vi "Pick&Place_ladder_shih_v6_center.vi"() -> ()   [LabVIEW 2016]
uses:
  WTF is this.ctl
  Classes/Controllers/I-O/Copy of NI-DAQ Folder/NI-DAQ.lvclass
  D:/INTT/V1/Classes/Controllers/I-O/Copy of I-O Folder/I-O.lvclass
  Classes/Controllers/Dispenser/Copy of Ultimus V2 Folder/Ultimus V2.lvclass
  <vilib>/Analysis/coordinate.llb/2D Cartesian Coordinate Rotation (Scalar).vi
  <vilib>/Utility/file.llb/Read Delimited Spreadsheet (DBL).vi
  <vilib>/Utility/file.llb/Write Delimited Spreadsheet (DBL).vi
  Classes/Controllers/Motion/Copy of Motion Folder/Motion.lvclass
  Classes/Controllers/Camera/Copy of Controller Folder/Controller.lvclass
  <vilib>/Analysis/NI_AALPro.lvlib
  Classes/Controllers/I-O/Copy of I-O Folder/I-O.lvclass
panel:
  in  "offset":dbl[][](array[numeric])=[[0.0, 0.0, 0.0, 0.0], [0.0, 0.0, 0.0, 0.0]]
  out "HPoS_CT":dbl[][](array[numeric]) format="%#_8g"
  out "chip distance by OGP":dbl format="%#_8g"
  out "displacement":dbl[](array[numeric])
  out "gantry position test":dbl[](array[numeric])
  out "stave target position":dbl[](array[numeric])
  out "chip distance by gantry":dbl format="%#_8g"
  out "after SL":dbl[](array[numeric]) format="%#_8g"
  out "after SR":dbl[](array[numeric]) format="%#_8g"
  out "after NL":dbl[](array[numeric]) format="%#_8g"
  out "S chip":dbl[](array[numeric]) format="%#_8g"
  out "N chip":dbl[](array[numeric]) format="%#_8g"
  in  "file path (dialog if empty) 2":path=path "C:/Users/PAGANIS/Desktop/shih cheng wei/OGP/test1-2.txt"
  out "bless from OGP !!! Center of  stave":dbl[](array[numeric])
  out "bless from OGP !! measured stave size":dbl[](array[numeric])
  in  "Bless from OGP":bool
  out "FROM Detail !!! Center of module on stave":dbl[](array[numeric])
  out "FROM Detail !! measured stave size":dbl[](array[numeric])
  in  "Align Stave in detail":bool
  in  "check height?":bool
  in  "Uttimus presssure":i64=10
  out "Status":bool
  out "measured HDI top-left position":dbl[][](array[numeric])
  in  "HDI vacuum channel":i32=18
  in  "vacuum":bool=TRUE
  in  "HDI vacuum":bool
  out "measured stave size":dbl[](array[numeric])
  out "Stave mark":dbl[][](array[numeric])
  out "Center of module on stave":dbl[](array[numeric])
  out "Center of HDI from alignment mark":dbl[](array[numeric])
  out "Measured HDI size":dbl[][](array[numeric])
  out "module positions on stave":T1[][](array[typedef])
  in  "Default Stave dimension":dbl[](array[numeric])=[34.0, 472.0, -0.335295, -0.000320234]
  in  "Default Stave upper left mark":dbl[](array[numeric])=[584.376, 675.576, 70.9882, 0.000840064]
  out "Needle parking position":dbl[](array[numeric])
  in  "Uppler / Lower Stave":bool=TRUE
  out "Gantry current position":dbl[](array[numeric])
  in  "READ Position":bool
  in  "Needle Height Compenstation\n(glue gap)":dbl=0.33
  in  "Needle Alignment":bool
  in  "Parking position":dbl[](array[numeric])=[625.0, 625.0, 0.0, 0.01]
  in  "GOTO":bool
  in  "Default Pickup Tool Position":dbl[][](array[numeric])=[[152.226, 682.729, 36.8129, -0.0151898], [700.0, 800.0, 20.0, 0.01]]
  in  "Number of module \nto be assembled":i32=1
  in  "Default HDI alignment \nmark position":dbl[](array[numeric])=[448.322, 976.582, 74.9872, 0.000191129]
  in  "Default HDI size":dbl[](array[numeric])=[24.2437, 231.446, -0.099339, 0.000191129]
  out "# of tasks excuted":i32
  out "HDI center positions":dbl[][](array[numeric])
  out "PickupTool \nCenterPosition":dbl[](array[numeric])
  in  "Inititalize":bool
  in  "Pick and place":bool
  in  "Deposit Glue":bool
  in  "Measure Pickup Tools":bool
  in  "Align Stave":bool
  out "default module position on stave":dbl[][](array[numeric])
  in  "Stop":bool
  in  "Measure HDI":bool
  # "Ladder Assembly"
  # "Lower\nmodule"
  # "Upper\nmodule"
  # "+"
  # "="
  # "Sensor 0.32 -> 200 micron glue thickness\nChips 0.37-> 140 micron glue thickness"
  # "ACTIONS"
  # "Stave infomation"
  # "theta had *-1"
  # "Module infomation"
  # "Pick and Place"
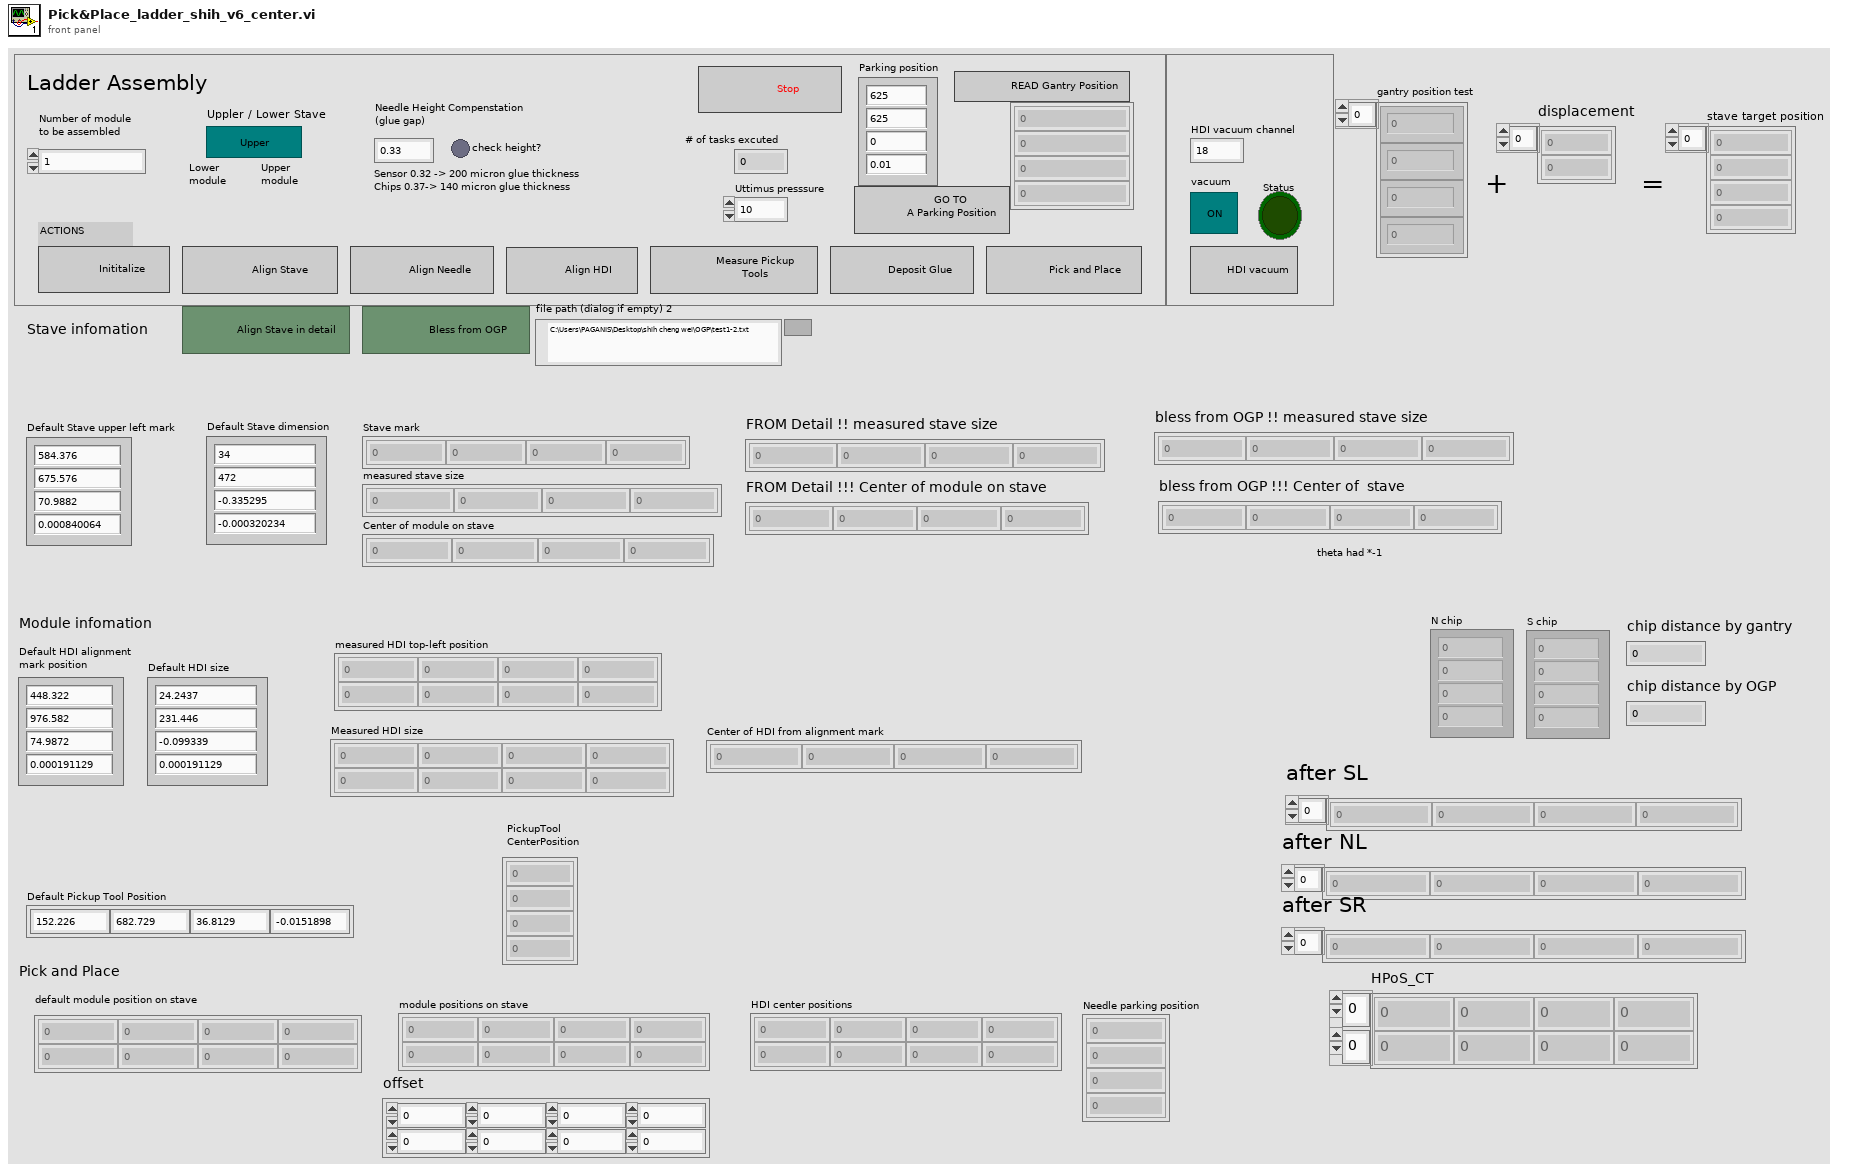
[diagram p1: front panel]
types:
  T1 = typedef "WTF is this.ctl" = dbl
  T2 = typedef "Controller.lvclass/Controllers.ctl" = cluster{"Copy of Motion.lvclass":refnum<class "Motion.lvclass">, "Copy of I-O.lvclass":refnum<class "I-O.lvclass">, "Copy of Dispenser.lvclass":refnum<class "Dispenser.lvclass">}
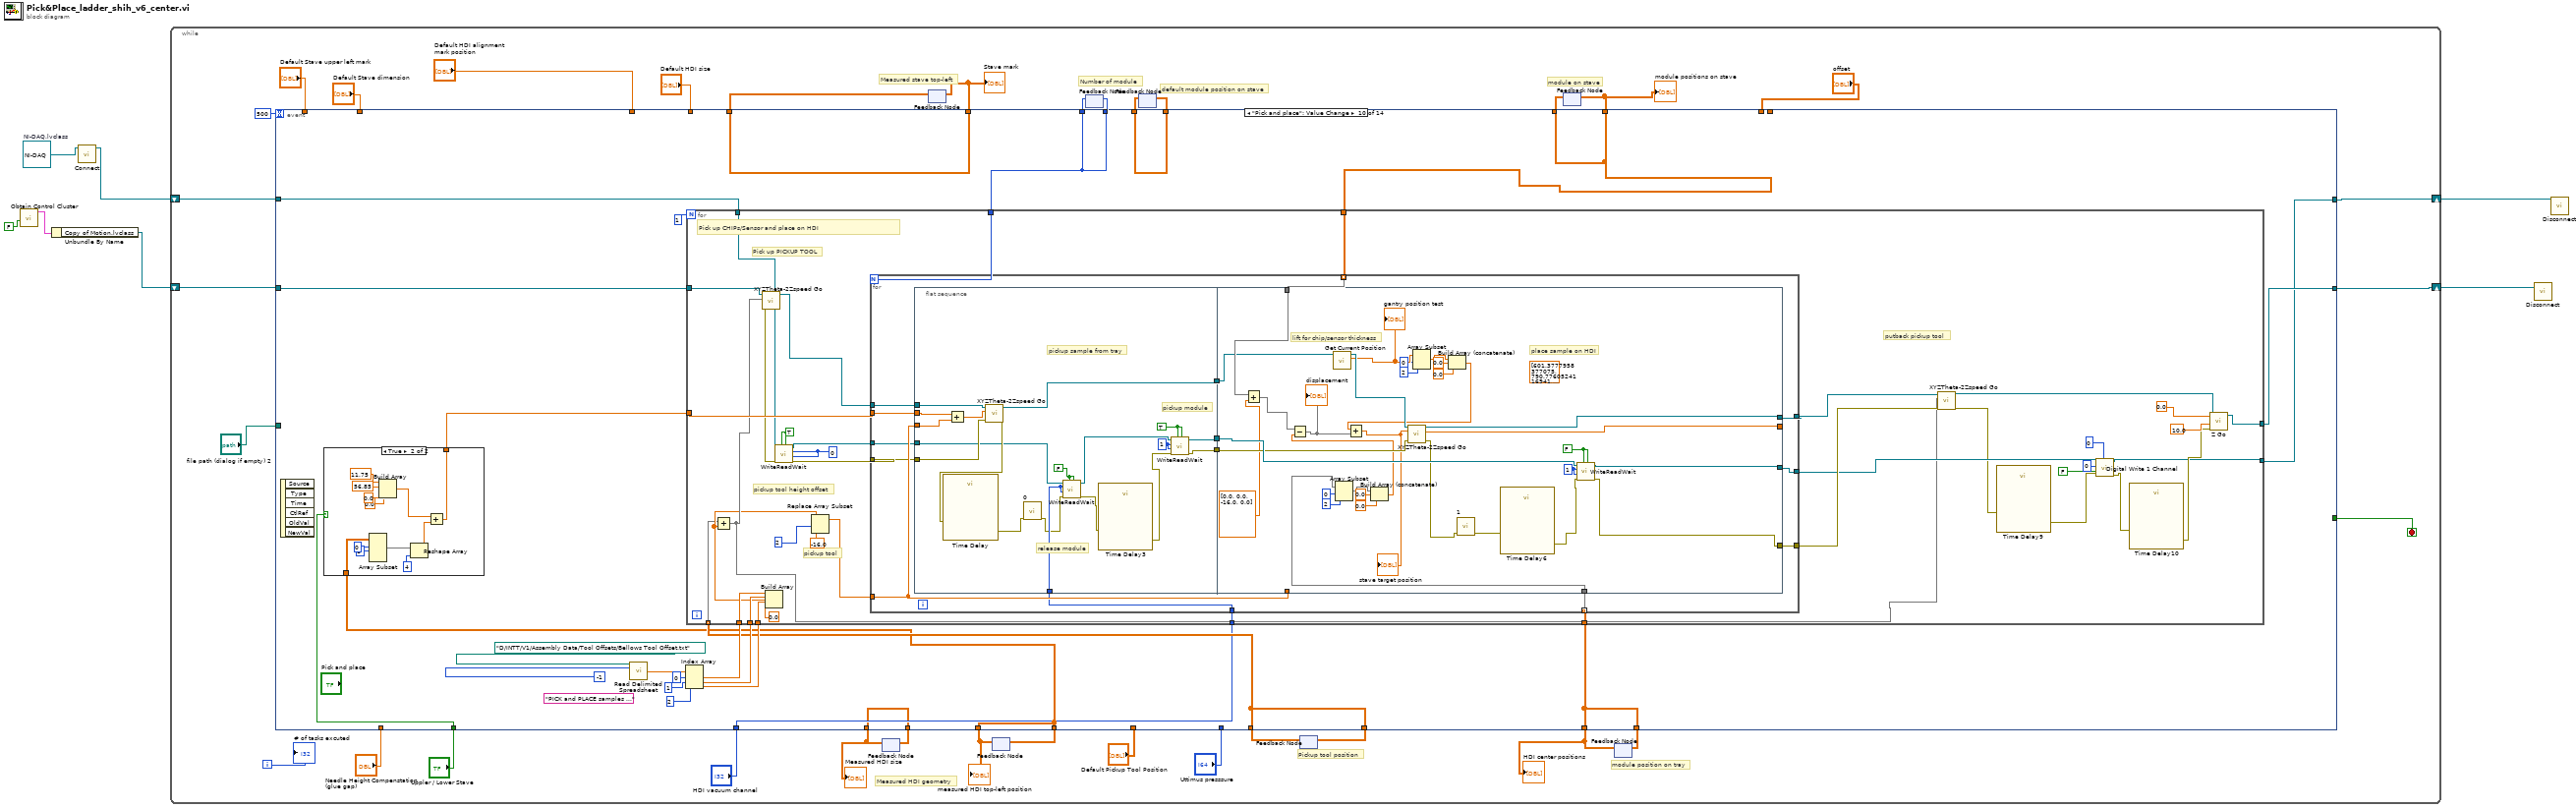
[diagram p0: block diagram]
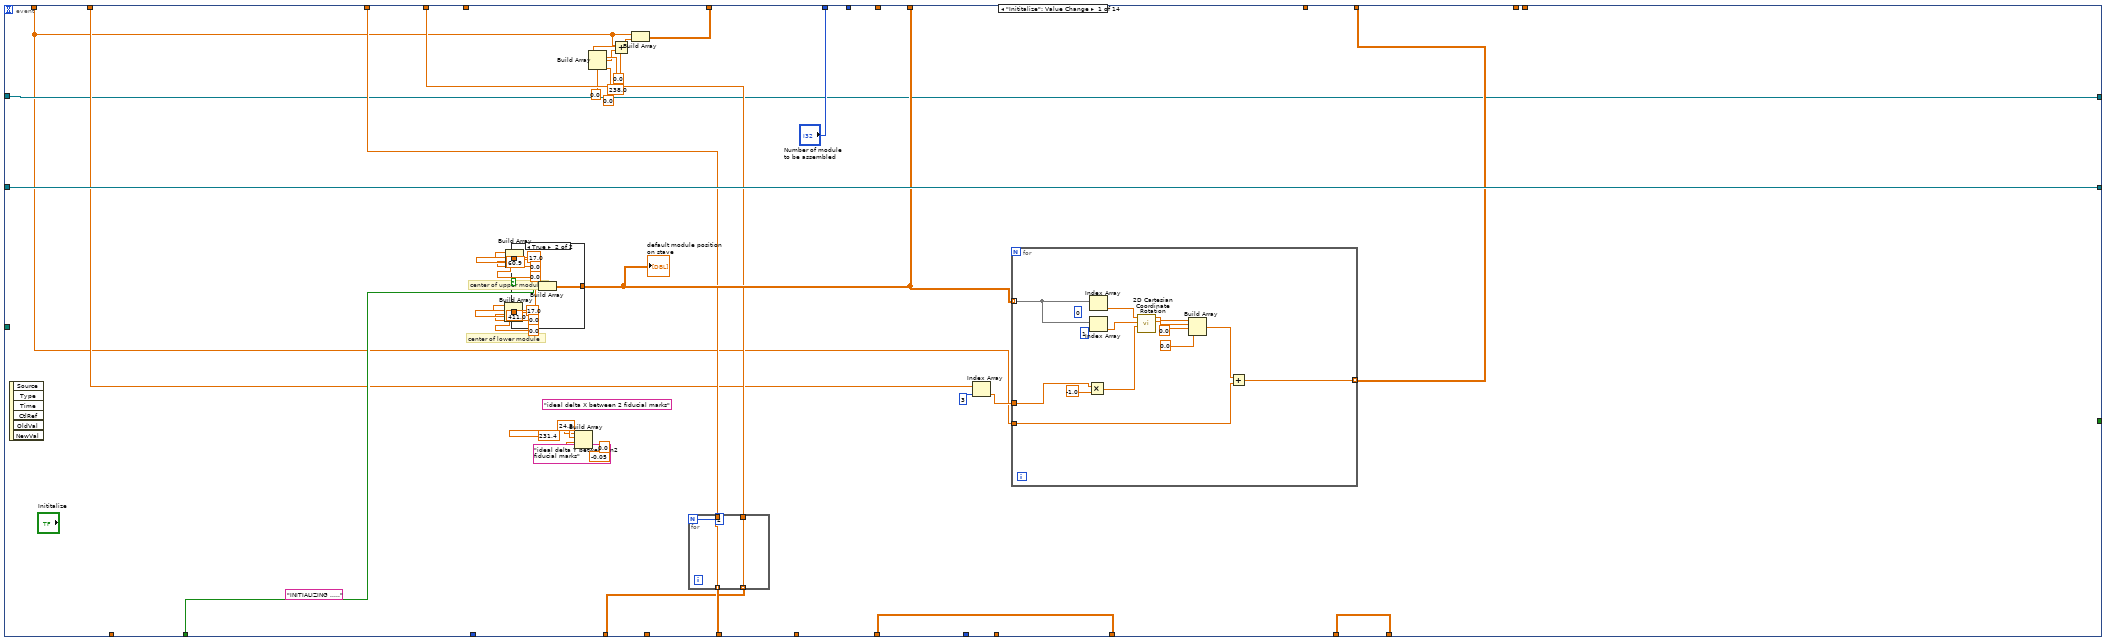
[diagram p2: hidden frame]
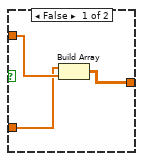
[diagram p3: hidden frame]
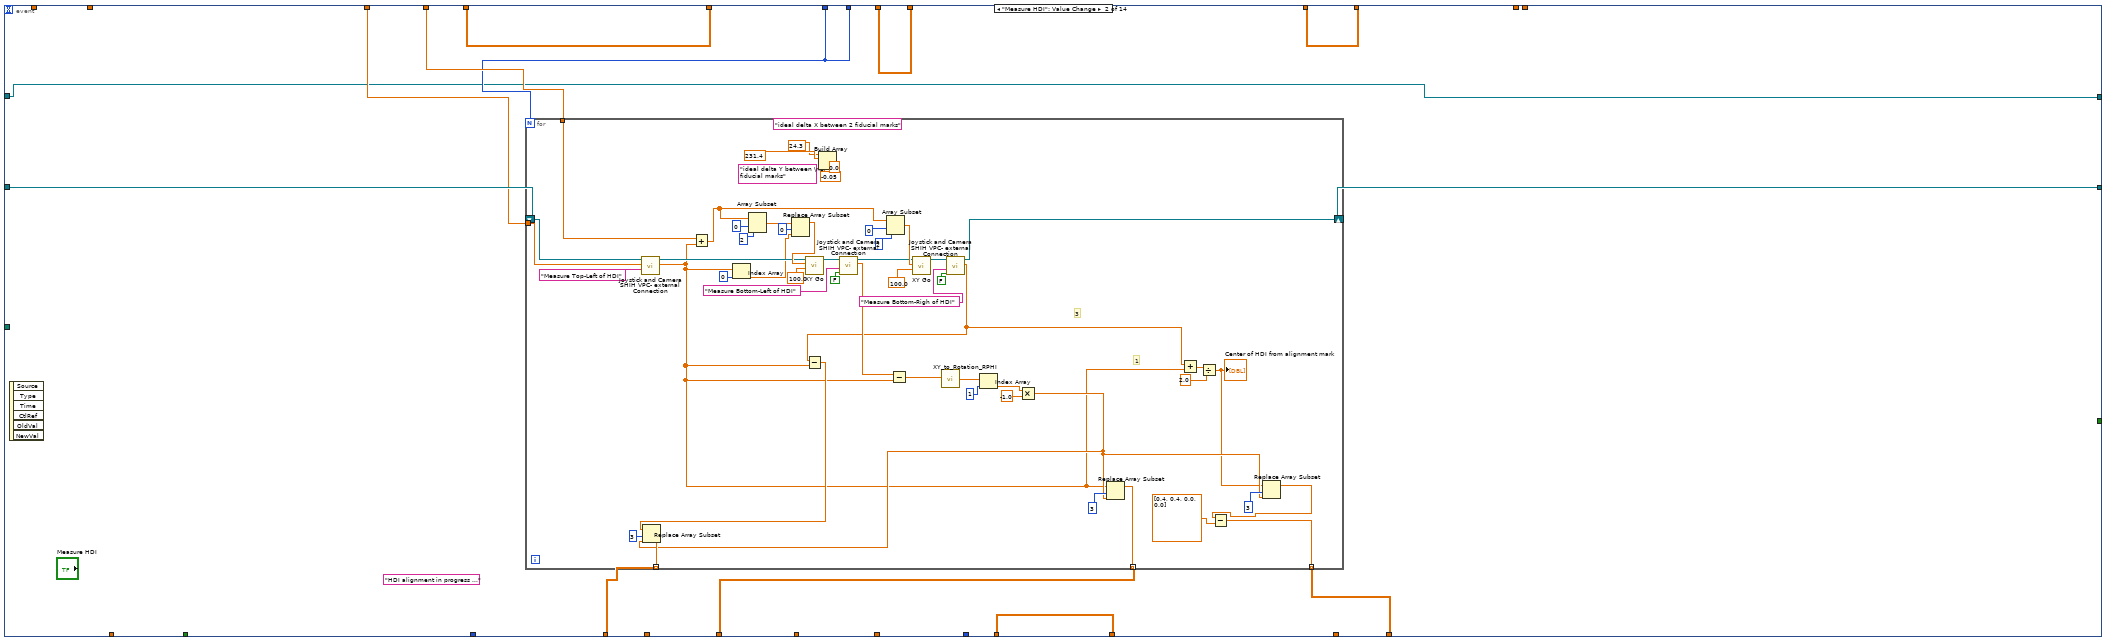
[diagram p4: hidden frame]
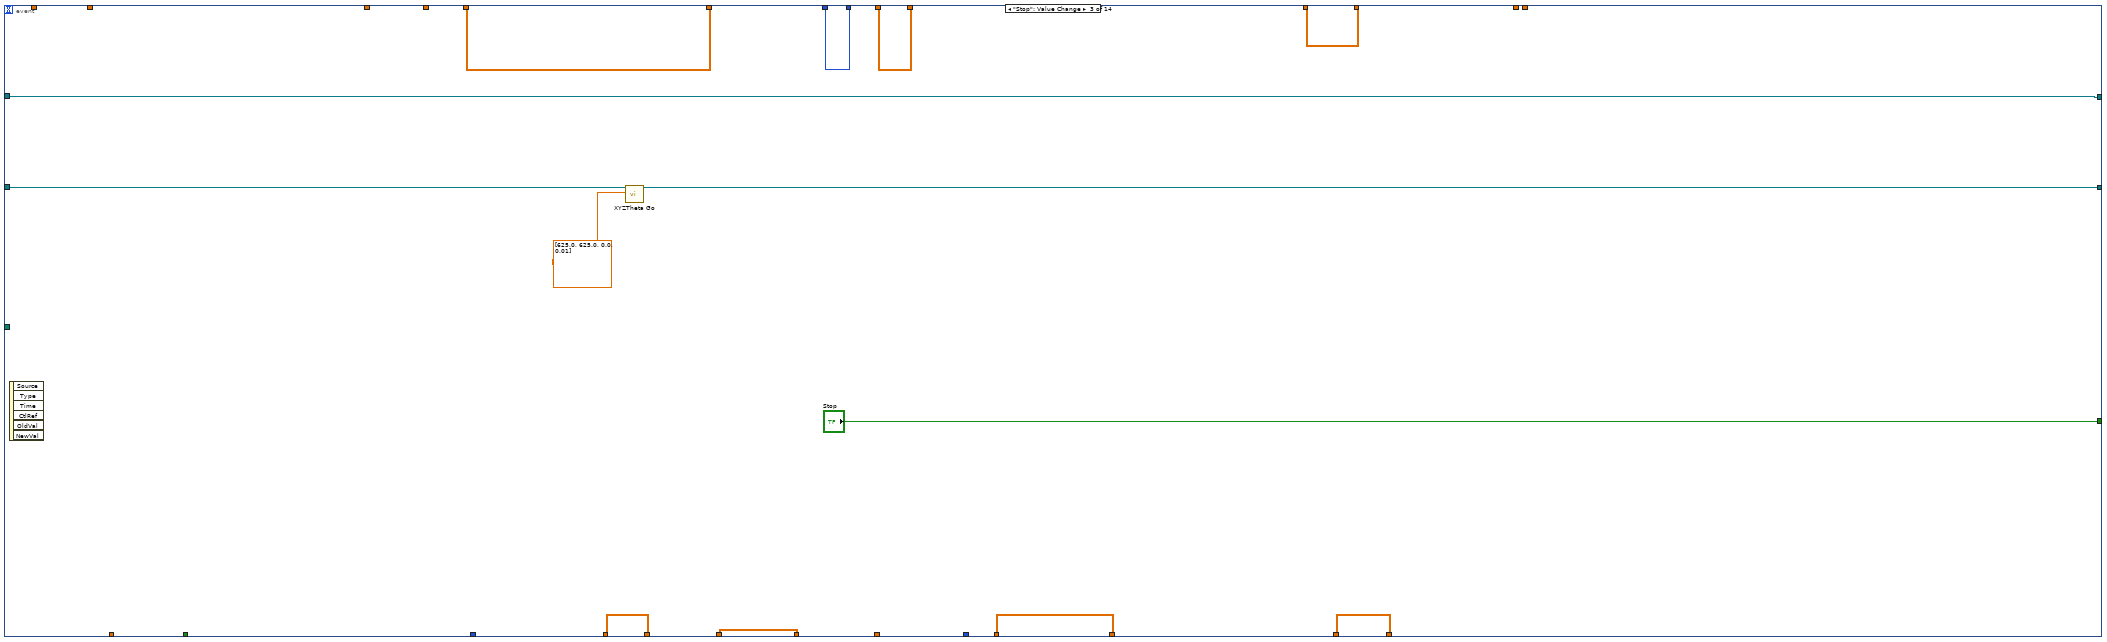
[diagram p5: hidden frame]
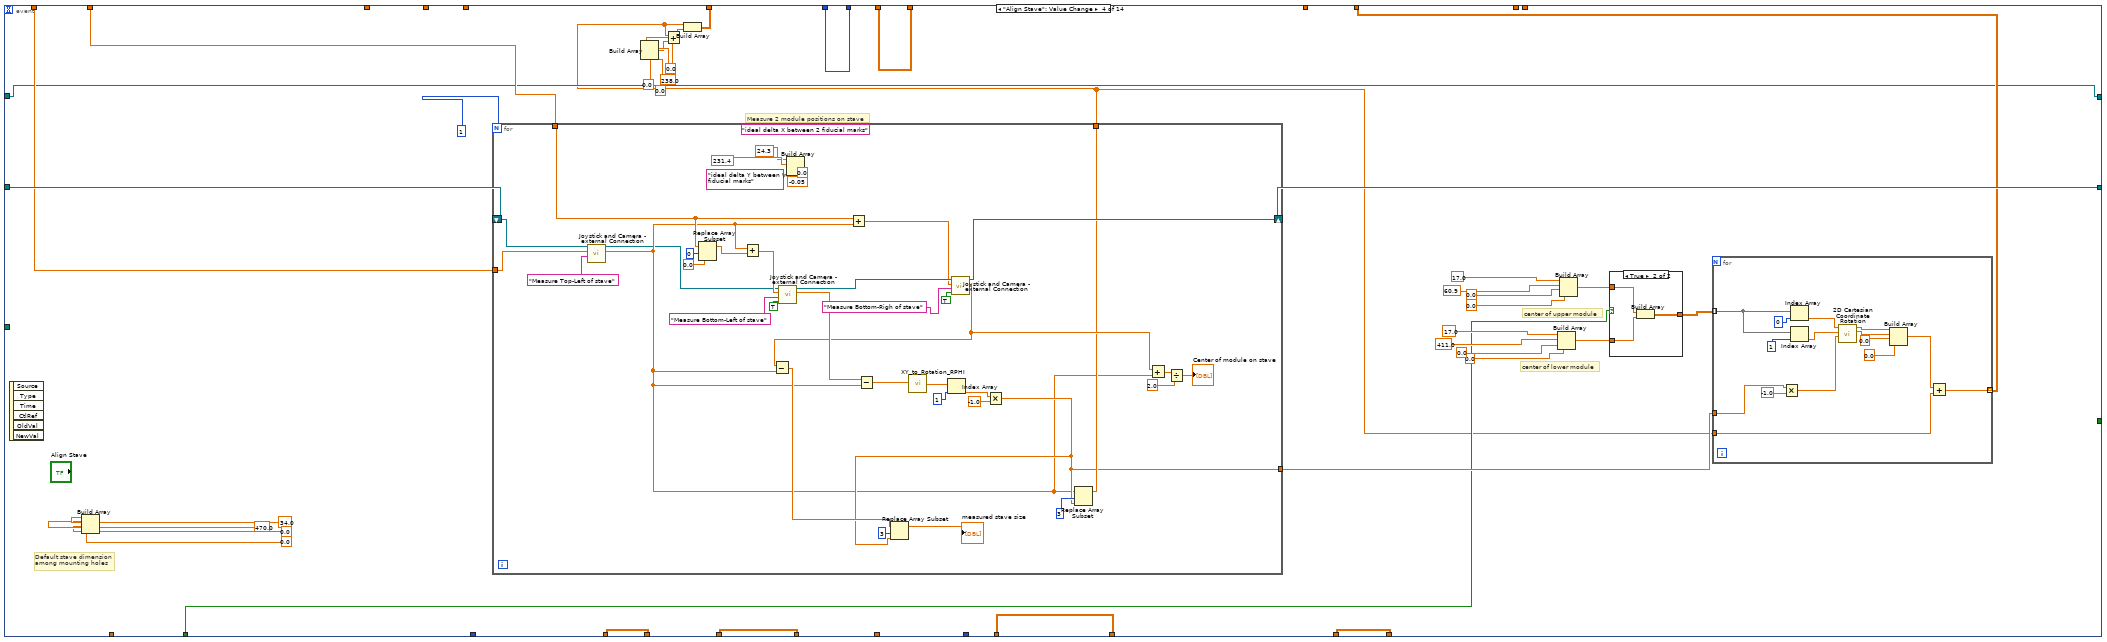
[diagram p6: hidden frame]
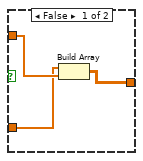
[diagram p7: hidden frame]
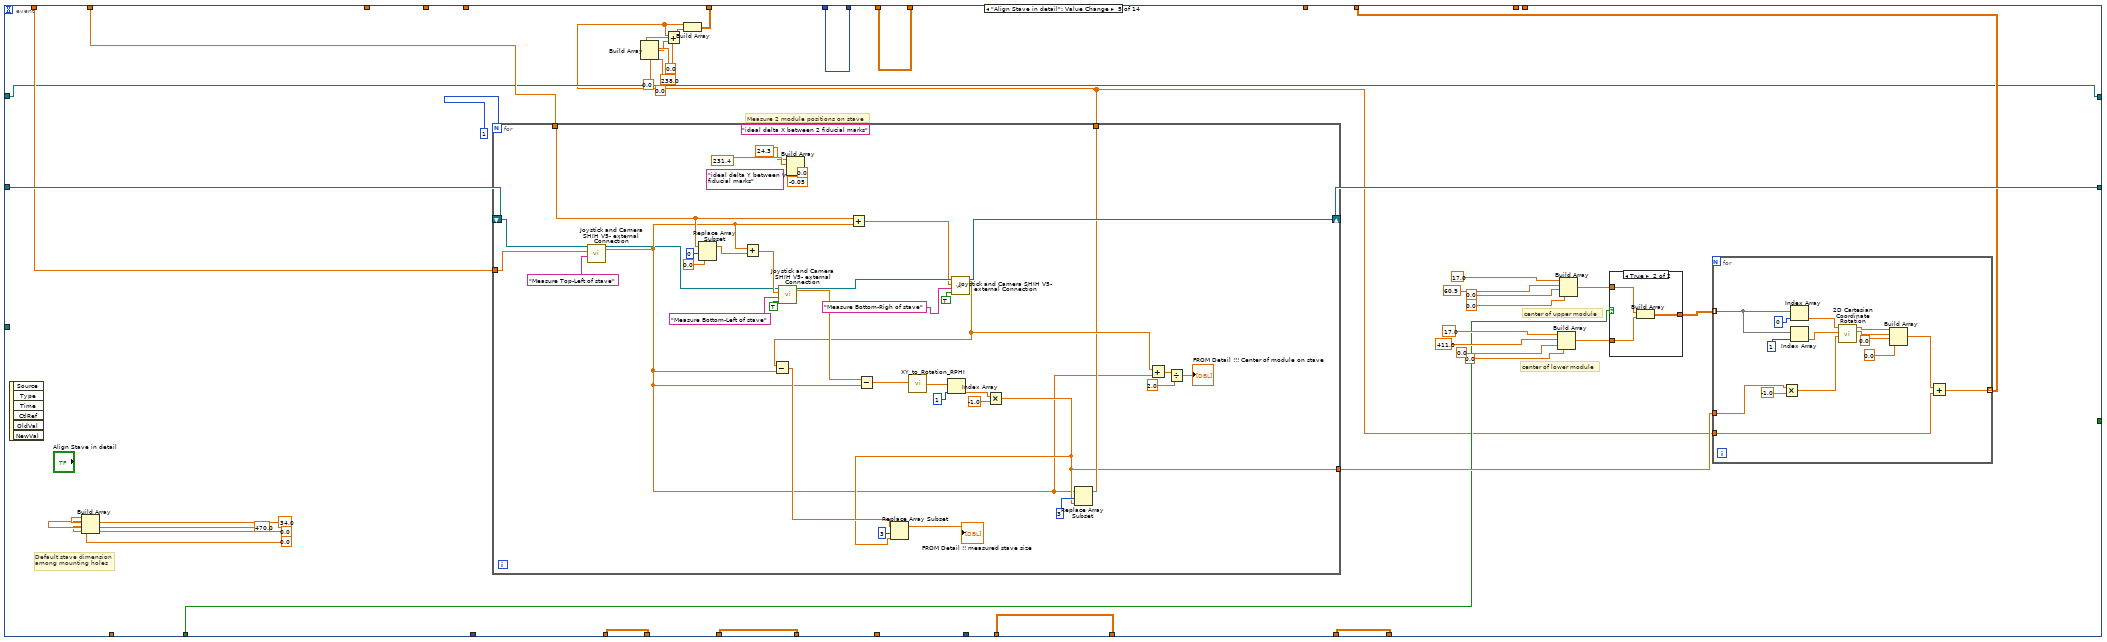
[diagram p8: hidden frame]
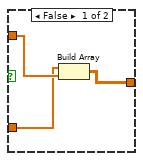
[diagram p9: hidden frame]
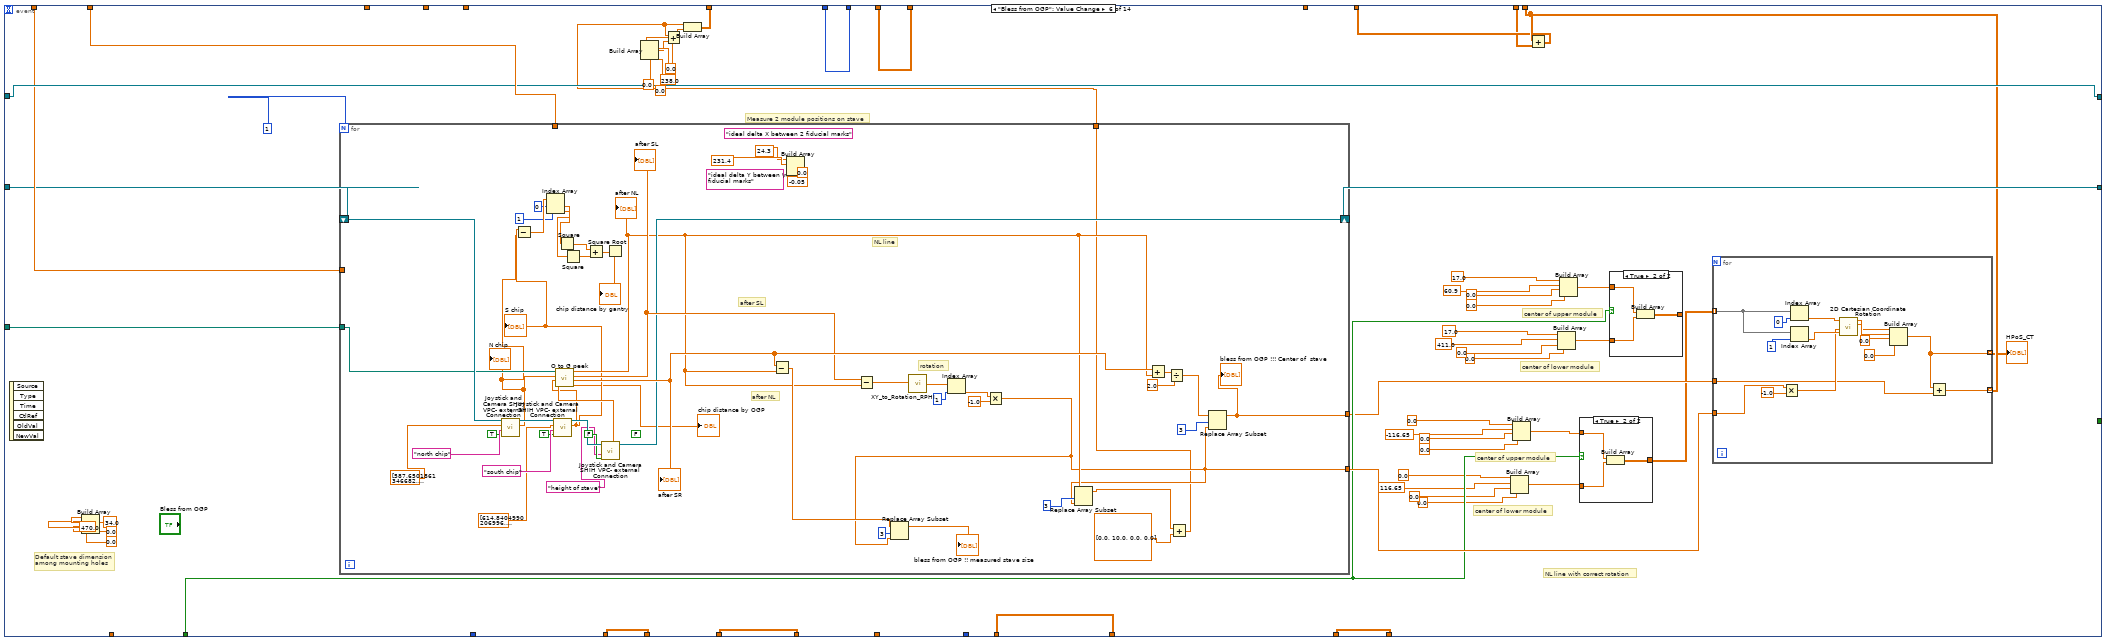
[diagram p10: hidden frame]
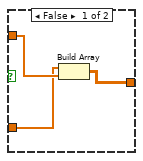
[diagram p11: hidden frame]
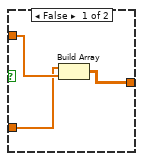
[diagram p12: hidden frame]
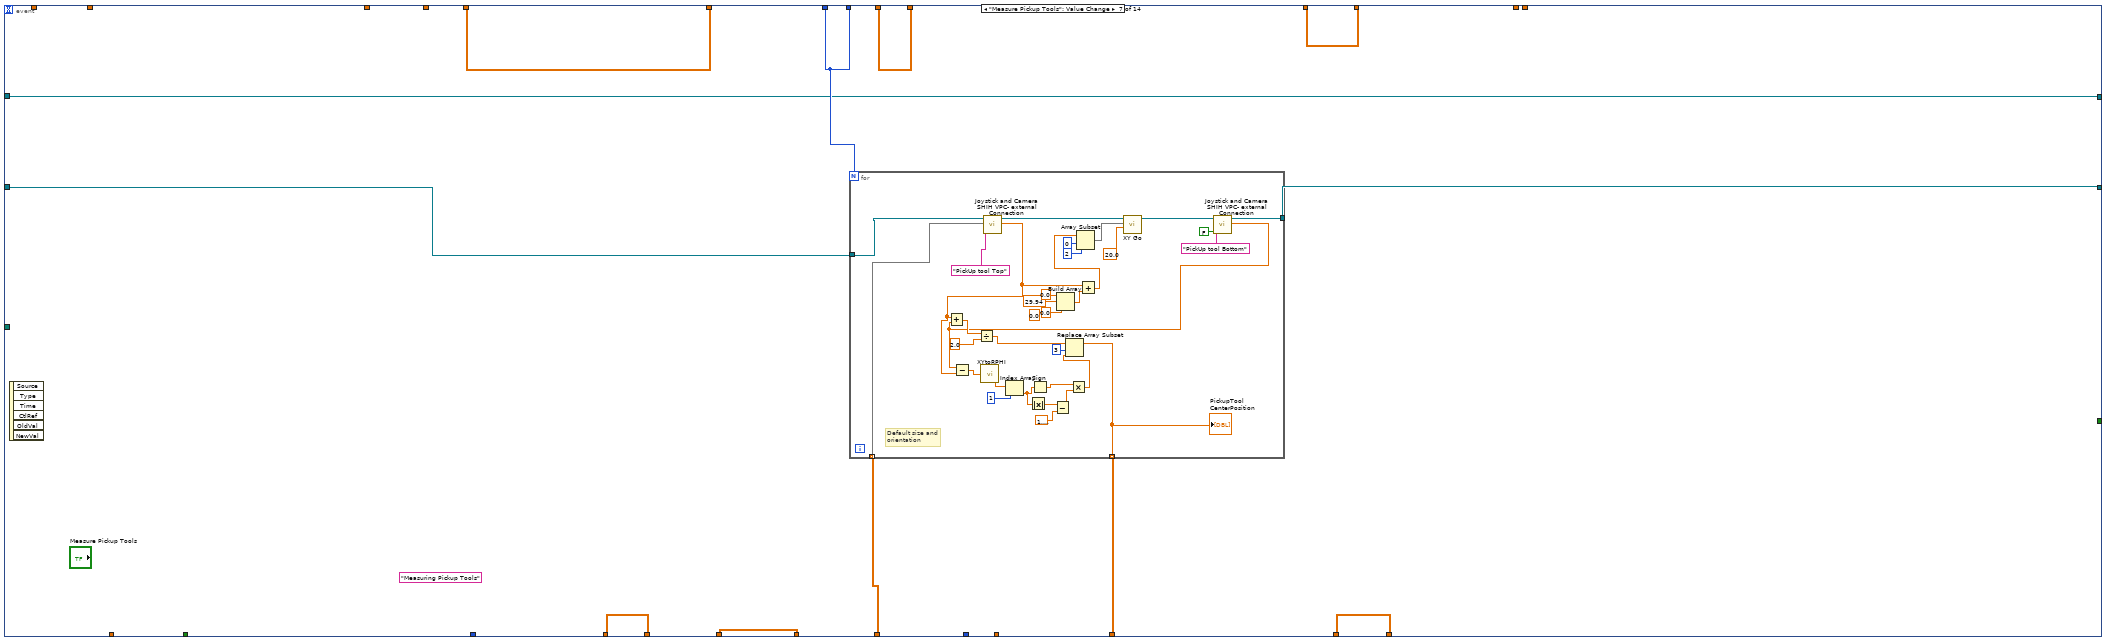
[diagram p13: hidden frame]
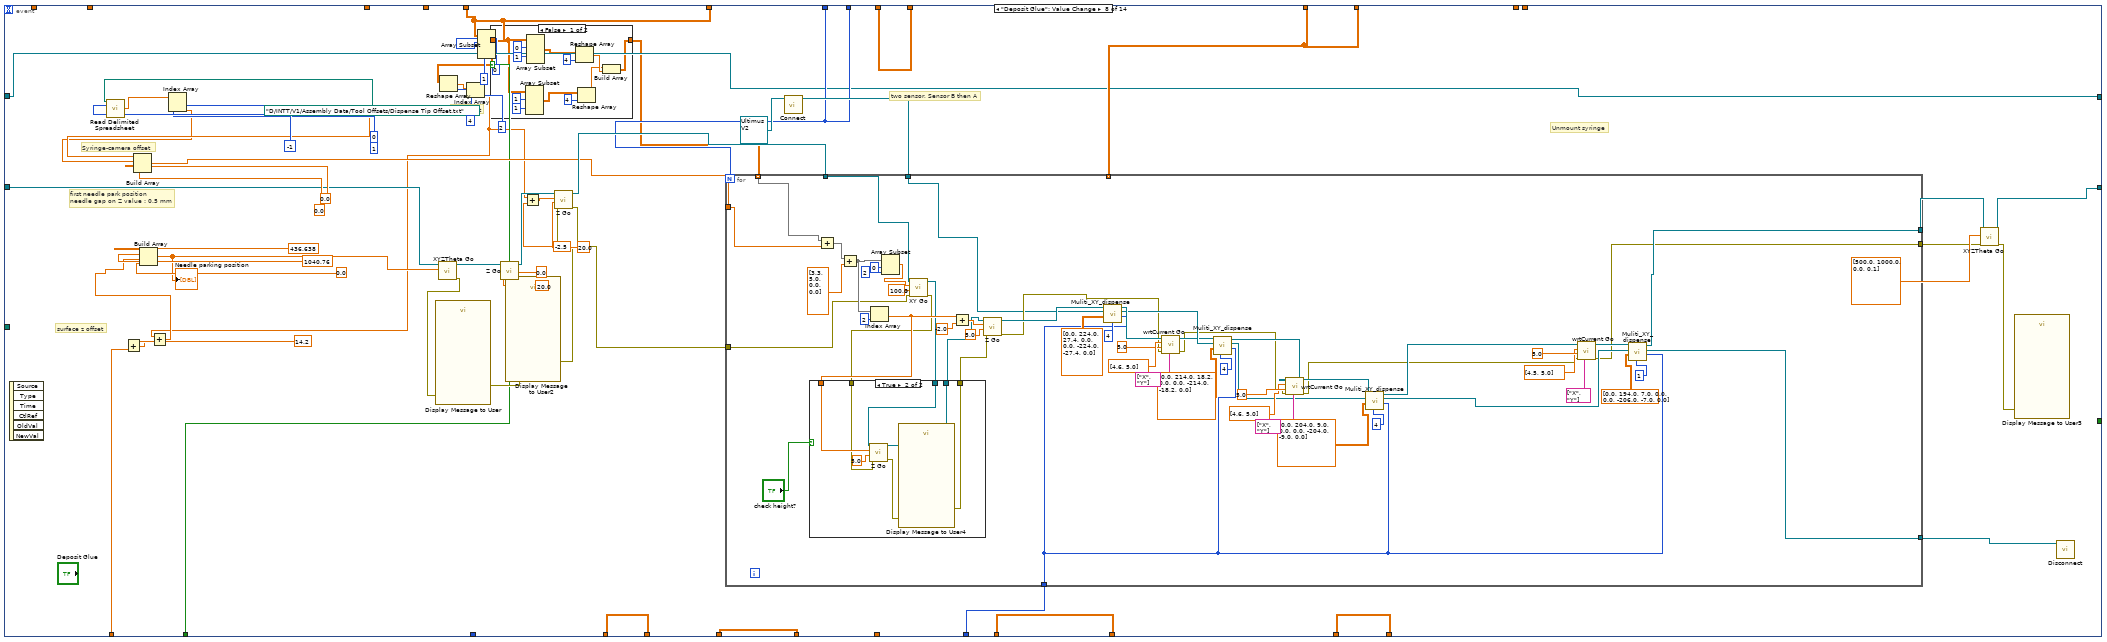
[diagram p14: hidden frame]
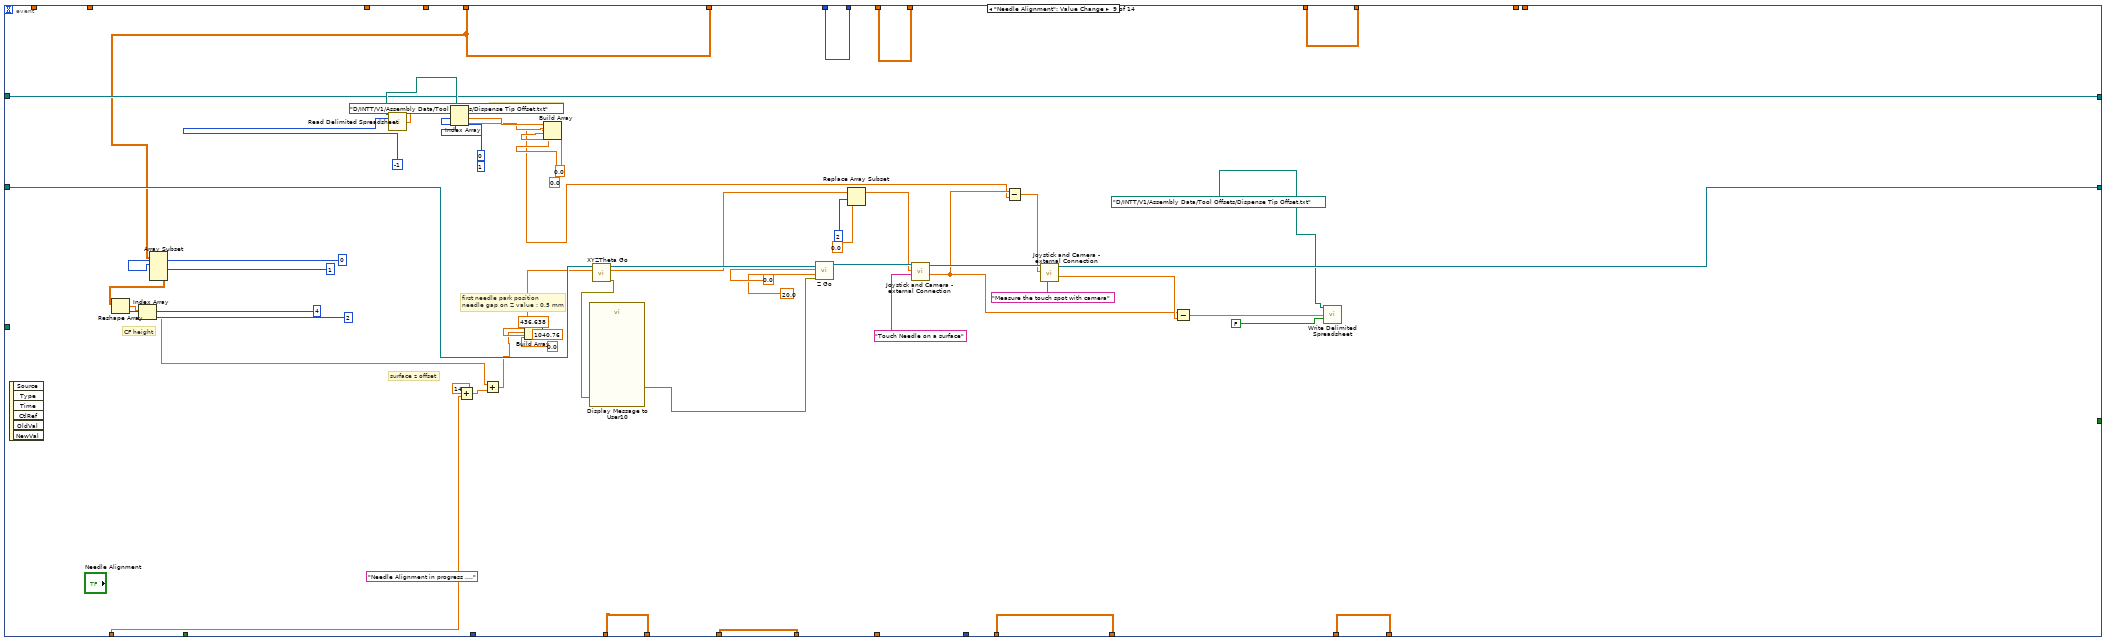
[diagram p17: hidden frame]
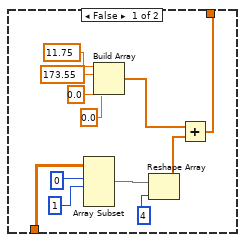
[diagram p18: hidden frame]
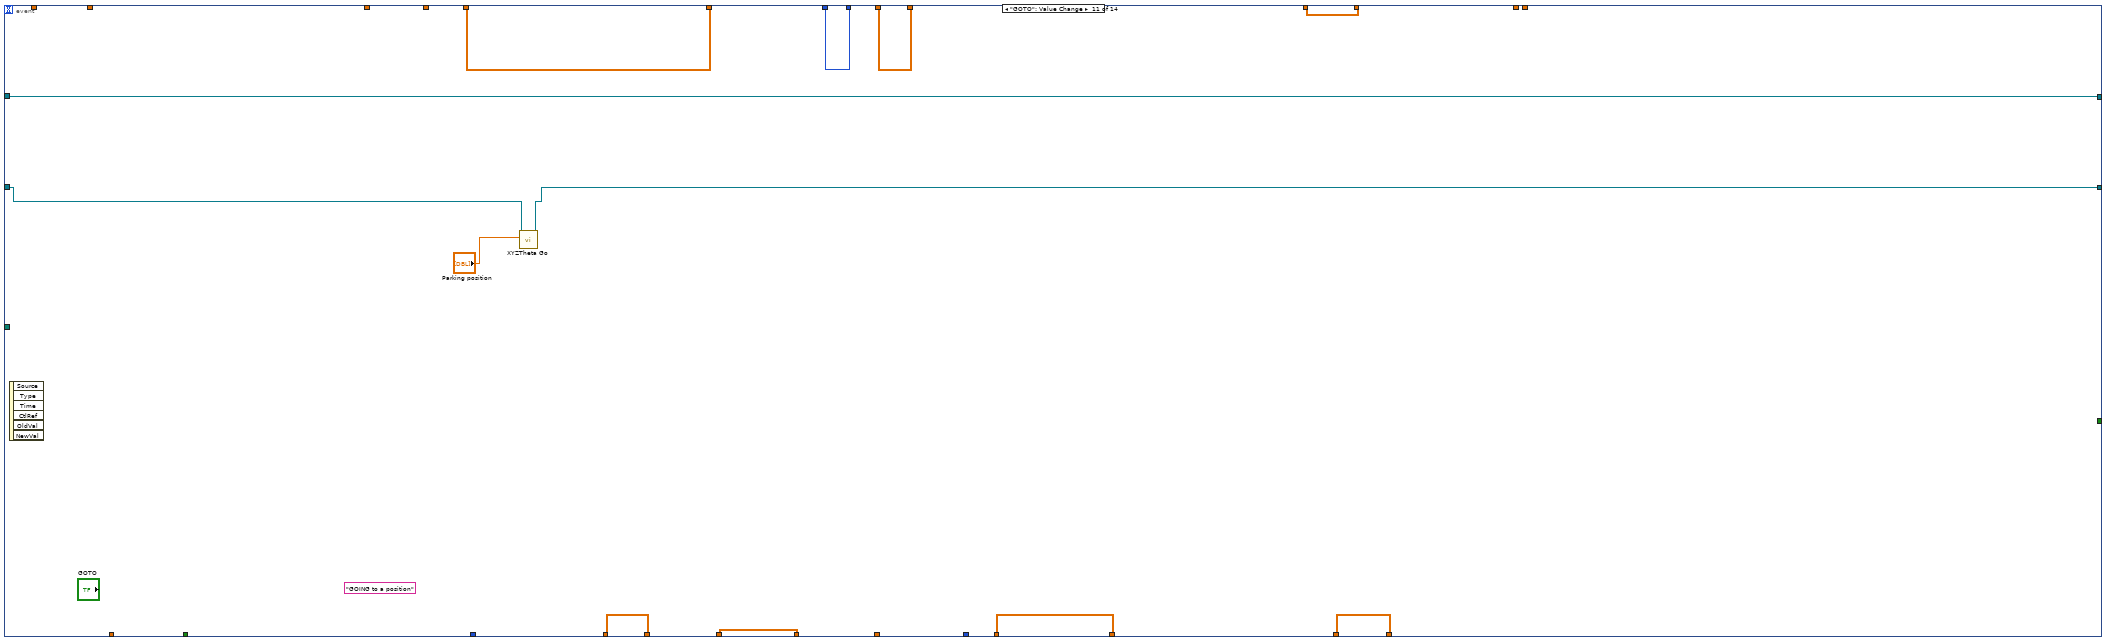
[diagram p19: hidden frame]
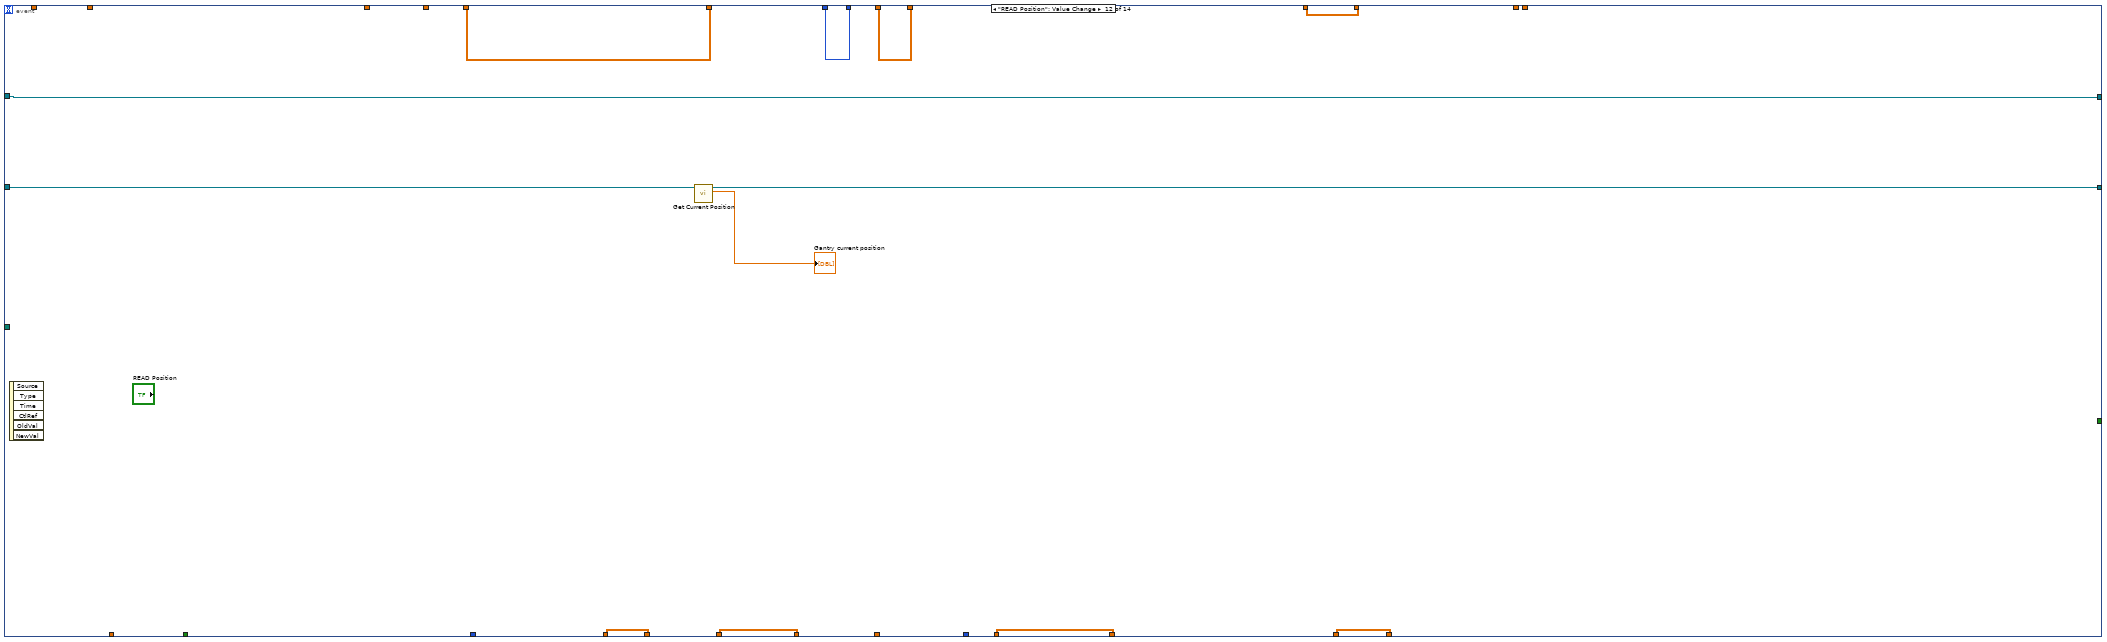
[diagram p20: hidden frame]
diagram:
  (unwired) T1[][] [[601.3777958377075, 790.7760524116941, 70.79103635532967, 0.0006918792394300775], [601.2163804240265, 1024.075996571705, 70.79103635532967, 0.0006918792394300775]] ("module positions on stave")
  w3 = refnum<class "NI-DAQ.lvclass"> refnum  # NI-DAQ.lvclass
  n1 = call "Obtain Control Cluster.vi"("I/O"=FALSE) -> ("Control Out"=w7:T2)  [unwired: 10 in]
  n2 = Unbundle By Name(w7) -> ("Copy of Motion.lvclass"=w5:refnum<class "Motion.lvclass">)
  n3 = call-dynamic "Connect.vi"("NI-DAQ in"=w3) -> ("NI-DAQ out"=w2:refnum<class "NI-DAQ.lvclass">)  [unwired: 9 in, 1 out]
  n4 = while {
    shift-right: [w34] -> w4
    shift-left: w5 -> [w41]
    shift-right: [w13] -> w1
    shift-left: w2 -> [w17]
    i -> [w33]
    stop <- w40 stop-if-true
    # "default module position on stave"
    # "Pickup tool position"
    # "Number of module"
    # "Measured HDI geometry"
    # "module position on tray"
    # "Measured stave top-left"
    # "module on stave"
    n5 = feedback #1() -> (w38:dbl[][])  [unwired: 1 in]
    n6 = feedback #2() -> (w39:dbl[][])  [unwired: 1 in]
    n7 = feedback #3() -> (w14:dbl[][])  [unwired: 1 in]
    n8 = feedback #4() -> (w32:i32)  [unwired: 1 in]
    n9 = feedback #5() -> (w27:dbl[][])  [unwired: 1 in]
    n10 = feedback #6() -> (w35:dbl[][])  [unwired: 1 in]
    n11 = feedback #7() -> (w21:dbl[][])  [unwired: 1 in]
    n12 = feedback #8() -> (w25:dbl[][])  [unwired: 1 in]
    "HDI center positions" <- w25
    n13 = event shown="[9] \"Pick and place\": Value Change" {
      selector: _ -> [_ _ _ _ _ _ _ _ _ _ _ _ _ _]
      dyn-events: _ -> [_ _ _ _ _ _ _ _ _ _ _ _ _ _]
      timeout: 500 -> [_ _ _ _ _ _ _ _ _ _ _ _ _ _]
      tunnel: w41 -> [w75 w114 w178 w208 w304 w388 w513 w586 w720 w764 w897 w915 w917 w938]
      tunnel: [_ _ "Stop" _ _ _ _ _ _ _ _ _ _ _] -> w40
      tunnel: [w42 w108 w173 w179 w275 w391 w508 w548 w686 w743 w903 w911 w925 w937] -> w18
      tunnel: w39 -> [_ w108 w173 _ _ _ w508 w548 w686 w743 w903 w911 w925 w937]
      tunnel: [w52 w106 w172 w204 w300 w413 w507 w572 w723 w746 w900 w910 w919 w935] -> w19
      tunnel: w38 -> [_ _ w172 w204 w300 w413 w507 w572 w723 w746 w900 w910 w919 w935]
      tunnel: w32 -> [_ w104 w175 w209 w305 w416 w504 w575 w725 w750 w902 w912 w923 w930]
      tunnel: [w57 w105 w170 w211 w307 w418 w506 w574 w721 w741 w898 w908 w921 w932] -> w37
      tunnel: w25 -> [w57 _ w170 w211 w307 w418 w506 w574 w721 w741 w898 w908 w921 w932]
      tunnel: [w73 w109 w171 w216 w312 w423 w512 w573 w722 w753 w899 w909 w920 w933] -> w36
      tunnel: w35 -> [_ w109 w171 w216 w312 w423 _ w573 w722 w753 w899 w909 w920 w933]
      tunnel: [w75 w113 w176 w205 w301 w414 w511 w576 w712 w754 w895 w914 w917 w938] -> w34
      tunnel: ["Number of module \nto be assembled" w104 w175 w209 w305 w416 w504 w575 w725 w750 w902 w912 w923 w930] -> w31
      tunnel: "Default HDI alignment \nmark position" -> [w55 w112 _ _ _ _ _ _ _ _ _ _ _ _]
      tunnel: "Default HDI size" -> [w54 w111 _ _ _ _ _ _ _ _ _ _ _ _]
      tunnel: [w62 w110 w174 w210 w306 w417 w509 w571 w724 w752 w901 w913 w924 w936] -> w28
      tunnel: w27 -> [_ w110 w174 w210 w306 w417 w509 w571 w724 w752 w901 w913 w924 w936]
      tunnel: "Default Pickup Tool Position" -> [w73 _ _ _ _ _ w510 _ _ _ _ _ _ _]
      tunnel: "Uppler / Lower Stave" -> [w58 _ _ w189 w285 w385 _ w556 _ w742 _ _ _ _]
      tunnel: "Default Stave upper left mark" -> [w43 _ _ w207 w303 w390 _ _ _ _ _ _ _ _]
      tunnel: "Default Stave dimension" -> [w51 _ _ w206 w302 w415 _ _ _ _ _ _ _ _]
      tunnel: [w59 w107 w168 w188 w284 w386 w505 w570 w703 w740 w893 w905 w922 w931] -> w20
      tunnel: w21 -> [_ w107 w168 _ _ _ w505 w570 w703 w740 w893 w905 w922 w931]
      tunnel: w17 -> [w50 w102 w166 w187 w283 w399 w502 w565 w701 w749 w892 w904 w929 w941]
      tunnel: [w50 w102 w166 w187 w283 w399 w502 w565 w701 w748 w892 w904 w916 w939] -> w13
      tunnel: "HDI vacuum channel" -> [_ _ _ _ _ _ _ _ _ w747 _ _ w926 w940]
      tunnel: [w53 w103 w167 w203 w299 w412 w503 w566 w702 w745 w894 w906 w918 w934] -> w15
      tunnel: w14 -> [_ _ w167 w203 w299 w412 w503 w566 w702 w745 w894 w906 w918 w934]
      tunnel: "Needle Height Compenstation\n(glue gap)" -> [_ _ _ _ _ _ _ w558 w694 _ _ _ _ _]
      tunnel: "Uttimus presssure" -> [_ _ _ _ _ _ _ w557 _ _ _ _ _ _]
      tunnel: "file path (dialog if empty) 2" -> [_ _ _ _ _ w389 _ _ _ _ _ _ _ _]
      tunnel: [_ _ _ _ _ w387 _ _ _ _ _ _ _ _] -> _
      tunnel: "offset" -> [_ _ _ _ _ w371 _ _ _ _ _ _ _ _]
      event "Inititalize": Value Change {
        (unwired) "INITIALIZING ....." ("String")
        (unwired) "ideal delta Y between \n2 fiducial marks"
        (unwired) "ideal delta X between 2 fiducial marks"
        # "center of lower module"
        # "center of upper module"
        n14 = event-data() -> ()  [unwired: 1 in, 6 out]
        n15 = Build Array(17.0 ("element"), 411.0 ("element"), 0.0 ("element"), 0.0 ("element")) -> (w63:dbl[])
        n16 = Build Array(17.0 ("element"), 60.9 ("element"), 0.0 ("element"), 0.0 ("element")) -> (w64:dbl[])
        n17 = case shown="True" w58 {
          tunnel: w64 -> [w84 w87]
          tunnel: w63 -> [w83 w86]
          tunnel: [w82 w85] -> w62
          frame False {
            n18 = Build Array(w83, w84) -> (w82:dbl[][])
          }
          frame True {
            n19 = Build Array(w87, w86) -> (w85:dbl[][])
          }
        }
        "default module position on stave" <- w62
        n20 = Build Array(24.3 ("y"), 231.4 ("y"), 0.0 ("element"), -0.05 ("element")) -> ()  [unwired: 1 out]
        n21 = Build Array(0.0 ("element"), 238.0 ("element"), 0.0 ("element"), 0.0 ("element")) -> (w45:dbl[])
        n22 = Add(x=w43, y=w45) -> (x+y=w44:dbl[])
        n23 = Build Array(w43, w44) -> (w42:dbl[][])
        n24 = for {
          N: 2 -> [_]
          tunnel: w55 -> [w81]
          tunnel: [w81] -> w53 mode=indexing
          tunnel: w54 -> [w80]
          tunnel: [w80] -> w52 mode=indexing
        }
        n25 = Index Array(array=w51, index=3) -> (element=w60:dbl)
        n26 = for {
          tunnel: w62 -> [w95] mode=indexing
          tunnel: w60 -> [w89]
          tunnel: w43 -> [w94]
          tunnel: [w92] -> w59 mode=indexing
          (unwired) 0 ("index")
          n27 = Multiply(x=w89, y=-1.0) -> (x*y=w90:dbl)
          n28 = Index Array(array=w95) -> (element=w98:dbl)  [unwired: 1 in]
          n29 = Index Array(array=w95, index=1) -> (element=w97:dbl)
          n30 = call-poly <vilib>:"2D Cartesian Coordinate Rotation.vi"("theta"=w90, "y"=w97, "x"=w98) -> ("y out"=w100:dbl, "x out"=w99:dbl)  [unwired: 6 in, 1 out]
          n31 = Build Array(w99, w100, 0.0 ("element"), 0.0 ("element")) -> (w93:dbl[])
          n32 = Add(x=w93, y=w94) -> (x+y=w92:dbl[])
        }
      }
      event "Measure HDI": Value Change {
        (unwired) "HDI alignment in progress ..." ("String")
        n33 = event-data() -> ()  [unwired: 1 in, 6 out]
        n34 = for {
          N: w104 -> [_]
          tunnel: w111 -> [w128]
          shift-right: [w125] -> w113
          shift-left: w114 -> [w126]
          tunnel: w112 -> [w127]
          tunnel: [w162] -> w103 mode=indexing
          tunnel: [w161] -> w106 mode=indexing
          tunnel: [w115] -> w105 mode=indexing
          (unwired) "ideal delta Y between \n2 fiducial marks"
          (unwired) "ideal delta X between 2 fiducial marks"
          # "1"
          # "3"
          n35 = call "Joystick and Camera SHIH VPC- external Connection.vi"("Motion in"=w126, "XYZTheta"=w127, "Measurement Point"="Measure Top-Left of HDI") -> ("Motion out"=w141:refnum<class "Motion.lvclass">, "Sum"=w118:dbl[])  [unwired: 4 in, 2 out]
          n36 = Add(x=w128, y=w118) -> (x+y=w145:dbl[])
          n37 = Index Array(array=w118, index=0) -> (element=w132:dbl)
          n38 = Array Subset(array=w145, index=0, length=2) -> (w144:dbl[])
          n39 = Replace Array Subset(array=w144, new element=w132, index=0) -> (w142:dbl[])
          n40 = call-dynamic "XY Go.vi"("Speed"=100.0, "XY"=w142, "Motion in"=w141) -> ("Motion out"=w149:refnum<class "Motion.lvclass">)  [unwired: 7 in, 1 out]
          n41 = Build Array(24.3 ("y"), 231.4 ("y"), 0.0 ("element"), -0.05 ("element")) -> ()  [unwired: 1 out]
          n42 = call "Joystick and Camera SHIH VPC- external Connection.vi"("Motion in"=w149, "Measurement Point"="Measure Bottom-Left of HDI", "Inital GO"=FALSE) -> ("Motion out"=w140:refnum<class "Motion.lvclass">, "Sum"=w131:dbl[])  [unwired: 4 in, 2 out]
          n43 = Array Subset(array=w145, index=0, length=2) -> (w155:dbl[])
          n44 = Subtract(x=w131, y=w118) -> (x-y=w139:dbl[])
          n45 = call-dynamic "XY Go.vi"("Speed"=100.0, "XY"=w155, "Motion in"=w140) -> ("Motion out"=w159:refnum<class "Motion.lvclass">)  [unwired: 7 in, 1 out]
          n46 = call "XY_to_Rotation_RPHI.vi"("X-Y"=w139) -> ("r-phi"=w135:dbl[])
          n47 = call "Joystick and Camera SHIH VPC- external Connection.vi"("Motion in"=w159, "Measurement Point"="Measure Bottom-Righ of HDI", "Inital GO"=FALSE) -> ("Motion out"=w125:refnum<class "Motion.lvclass">, "Sum"=w122:dbl[])  [unwired: 4 in, 2 out]
          n48 = Subtract(x=w122, y=w118) -> (x-y=w123:dbl[])
          n49 = Index Array(array=w135, index=1) -> (element=w129:dbl)
          n50 = Multiply(x=w129, y=-1.0) -> (x*y=w120:dbl)
          n51 = Replace Array Subset(array=w123, new element=w120, index=3) -> (w161:dbl[])
          n52 = Replace Array Subset(array=w118, new element=w120, index=3) -> (w162:dbl[])
          n53 = Add(x=w122, y=w118) -> (x+y=w164:dbl[])
          n54 = Divide(x=w164, y=2.0) -> (x/y=w119:dbl[])
          "Center of HDI from alignment mark" <- w119
          n55 = Replace Array Subset(array=w119, new element=w120, index=3) -> (w116:dbl[])
          n56 = Subtract(x=w116, y=dbl[] [0.4, 0.4, 0.0, 0.0]) -> (x-y=w115:dbl[])
        }
      }
      event "Stop": Value Change {
        n57 = event-data() -> ()  [unwired: 1 in, 6 out]
        n58 = call "XYZTheta Go.vi"("XYZTheta In"=dbl[] [625.0, 625.0, 0.0, 0.01], "Motion in"=w178) -> ("Motion out"=w176:refnum<class "Motion.lvclass">)  [unwired: 7 in, 2 out]
      }
      event "Align Stave": Value Change {
        # "center of lower module"
        # "center of upper module"
        # "Default stave dimension\namong mounting holes"
        # "Measure 2 module positions on stave"
        n59 = event-data() -> ()  [unwired: 1 in, 6 out]
        n60 = Build Array(34.0 ("element"), 470.0 ("element"), 0.0 ("element"), 0.0 ("element")) -> ()  [unwired: 1 out]
        n61 = for {
          N: 1 -> [_]
          tunnel: w206 -> [w223]
          shift-right: [w233] -> w205
          shift-left: w208 -> [w234]
          tunnel: w207 -> [w235]
          tunnel: [w228] -> w181
          tunnel: [w226] -> w191
          (unwired) "ideal delta Y between \n2 fiducial marks"
          (unwired) "ideal delta X between 2 fiducial marks"
          n62 = call "Joystick and Camera - external Connection.vi"("Motion in"=w234, "XYZTheta"=w235, "Measurement Point"="Measure Top-Left of stave") -> ("Motion out"=w217:refnum<class "Motion.lvclass">, "Sum"=w219:dbl[])  [unwired: 4 in, 2 out]
          n63 = Replace Array Subset(array=w223, new element=0.0 ("new element/subarray"), index=0) -> (w220:dbl[])
          n64 = Add(x=w219, y=w220) -> (x+y=w218:dbl[])
          n65 = call "Joystick and Camera - external Connection.vi"("Motion in"=w217, "XYZTheta"=w218, "Measurement Point"="Measure Bottom-Left of stave", "Inital GO"=TRUE) -> ("Motion out"=w225:refnum<class "Motion.lvclass">, "Sum"=w238:dbl[])  [unwired: 3 in, 2 out]
          n66 = Build Array(24.3 ("y"), 231.4 ("y"), 0.0 ("element"), -0.05 ("element")) -> ()  [unwired: 1 out]
          n67 = Add(x=w223, y=w219) -> (x+y=w224:dbl[])
          n68 = Subtract(x=w238, y=w219) -> (x-y=w244:dbl[])
          n69 = call "XY_to_Rotation_RPHI.vi"("X-Y"=w244) -> ("r-phi"=w240:dbl[])
          n70 = Index Array(array=w240, index=1) -> (element=w236:dbl)
          n71 = call "Joystick and Camera - external Connection.vi"("Motion in"=w225, "XYZTheta"=w224, "Measurement Point"="Measure Bottom-Righ of stave", "Inital GO"=TRUE) -> ("Motion out"=w233:refnum<class "Motion.lvclass">, "Sum"=w230:dbl[])  [unwired: 3 in, 2 out]
          n72 = Subtract(x=w230, y=w219) -> (x-y=w231:dbl[])
          n73 = Multiply(x=w236, y=-1.0) -> (x*y=w226:dbl)
          n74 = Replace Array Subset(array=w231, new element=w226, index=3) -> (→"measured stave size":dbl[])
          n75 = Replace Array Subset(array=w219, new element=w226, index=3) -> (w228:dbl[])
          n76 = Add(x=w230, y=w219) -> (x+y=w252:dbl[])
          n77 = Divide(x=w252, y=2.0) -> (x/y=→"Center of module on stave":dbl[])
        }
        n78 = Build Array(0.0 ("element"), 238.0 ("element"), 0.0 ("element"), 0.0 ("element")) -> (w182:dbl[])
        n79 = Add(x=w181, y=w182) -> (x+y=w180:dbl[])
        n80 = Build Array(w181, w180) -> (w179:dbl[][])
        n81 = Build Array(17.0 ("element"), 411.0 ("element"), 0.0 ("element"), 0.0 ("element")) -> (w193:dbl[])
        n82 = Build Array(17.0 ("element"), 60.9 ("element"), 0.0 ("element"), 0.0 ("element")) -> (w194:dbl[])
        n83 = case shown="True" w189 {
          tunnel: w194 -> [w271 w274]
          tunnel: w193 -> [w270 w273]
          tunnel: [w269 w272] -> w192
          frame False {
            n84 = Build Array(w270, w271) -> (w269:dbl[][])
          }
          frame True {
            n85 = Build Array(w274, w273) -> (w272:dbl[][])
          }
        }
        n86 = for {
          tunnel: w192 -> [w262] mode=indexing
          tunnel: w191 -> [w257]
          tunnel: w181 -> [w261]
          tunnel: [w259] -> w188 mode=indexing
          n87 = Multiply(x=w257, y=-1.0) -> (x*y=w256:dbl)
          n88 = Index Array(array=w262, index=0) -> (element=w265:dbl)
          n89 = Index Array(array=w262, index=1) -> (element=w264:dbl)
          n90 = call-poly <vilib>:"2D Cartesian Coordinate Rotation.vi"("theta"=w256, "y"=w264, "x"=w265) -> ("y out"=w267:dbl, "x out"=w266:dbl)  [unwired: 6 in, 1 out]
          n91 = Build Array(w266, w267, 0.0 ("element"), 0.0 ("element")) -> (w260:dbl[])
          n92 = Add(x=w260, y=w261) -> (x+y=w259:dbl[])
        }
      }
      event "Align Stave in detail": Value Change {
        # "center of lower module"
        # "center of upper module"
        # "Default stave dimension\namong mounting holes"
        # "Measure 2 module positions on stave"
        n93 = event-data() -> ()  [unwired: 1 in, 6 out]
        n94 = Build Array(34.0 ("element"), 470.0 ("element"), 0.0 ("element"), 0.0 ("element")) -> ()  [unwired: 1 out]
        n95 = for {
          N: 1 -> [_]
          tunnel: w302 -> [w319]
          shift-right: [w329] -> w301
          shift-left: w304 -> [w330]
          tunnel: w303 -> [w331]
          tunnel: [w324] -> w277
          tunnel: [w322] -> w287
          (unwired) "ideal delta Y between \n2 fiducial marks"
          (unwired) "ideal delta X between 2 fiducial marks"
          n96 = call "Joystick and Camera SHIH V5- external Connection.vi"("Motion in"=w330, "XYZTheta"=w331, "Measurement Point"="Measure Top-Left of stave") -> ("final out"=w315:dbl[], "Motion out"=w313:refnum<class "Motion.lvclass">)  [unwired: 5 in, 1 out]
          n97 = Replace Array Subset(array=w319, new element=0.0 ("new element/subarray"), index=0) -> (w316:dbl[])
          n98 = Add(x=w315, y=w316) -> (x+y=w314:dbl[])
          n99 = call "Joystick and Camera SHIH V5- external Connection.vi"("Motion in"=w313, "XYZTheta"=w314, "Measurement Point"="Measure Bottom-Left of stave", "Inital GO"=TRUE) -> ("final out"=w334:dbl[], "Motion out"=w321:refnum<class "Motion.lvclass">)  [unwired: 4 in, 1 out]
          n100 = Build Array(24.3 ("y"), 231.4 ("y"), 0.0 ("element"), -0.05 ("element")) -> ()  [unwired: 1 out]
          n101 = Add(x=w319, y=w315) -> (x+y=w320:dbl[])
          n102 = Subtract(x=w334, y=w315) -> (x-y=w340:dbl[])
          n103 = call "XY_to_Rotation_RPHI.vi"("X-Y"=w340) -> ("r-phi"=w336:dbl[])
          n104 = Index Array(array=w336, index=1) -> (element=w332:dbl)
          n105 = call "Joystick and Camera SHIH V5- external Connection.vi"("Motion in"=w321, "XYZTheta"=w320, "Measurement Point"="Measure Bottom-Righ of stave", "Inital GO"=TRUE) -> ("final out"=w326:dbl[], "Motion out"=w329:refnum<class "Motion.lvclass">)  [unwired: 4 in, 1 out]
          n106 = Subtract(x=w326, y=w315) -> (x-y=w327:dbl[])
          n107 = Multiply(x=w332, y=-1.0) -> (x*y=w322:dbl)
          n108 = Replace Array Subset(array=w327, new element=w322, index=3) -> (→"FROM Detail !! measured stave size":dbl[])
          n109 = Replace Array Subset(array=w315, new element=w322, index=3) -> (w324:dbl[])
          n110 = Add(x=w326, y=w315) -> (x+y=w348:dbl[])
          n111 = Divide(x=w348, y=2.0) -> (x/y=→"FROM Detail !!! Center of module on stave":dbl[])
        }
        n112 = Build Array(0.0 ("element"), 238.0 ("element"), 0.0 ("element"), 0.0 ("element")) -> (w278:dbl[])
        n113 = Add(x=w277, y=w278) -> (x+y=w276:dbl[])
        n114 = Build Array(w277, w276) -> (w275:dbl[][])
        n115 = Build Array(17.0 ("element"), 411.0 ("element"), 0.0 ("element"), 0.0 ("element")) -> (w289:dbl[])
        n116 = Build Array(17.0 ("element"), 60.9 ("element"), 0.0 ("element"), 0.0 ("element")) -> (w290:dbl[])
        n117 = case shown="True" w285 {
          tunnel: w290 -> [w367 w370]
          tunnel: w289 -> [w366 w369]
          tunnel: [w365 w368] -> w288
          frame False {
            n118 = Build Array(w366, w367) -> (w365:dbl[][])
          }
          frame True {
            n119 = Build Array(w370, w369) -> (w368:dbl[][])
          }
        }
        n120 = for {
          tunnel: w288 -> [w358] mode=indexing
          tunnel: w287 -> [w353]
          tunnel: w277 -> [w357]
          tunnel: [w355] -> w284 mode=indexing
          n121 = Multiply(x=w353, y=-1.0) -> (x*y=w352:dbl)
          n122 = Index Array(array=w358, index=0) -> (element=w361:dbl)
          n123 = Index Array(array=w358, index=1) -> (element=w360:dbl)
          n124 = call-poly <vilib>:"2D Cartesian Coordinate Rotation.vi"("theta"=w352, "y"=w360, "x"=w361) -> ("y out"=w363:dbl, "x out"=w362:dbl)  [unwired: 6 in, 1 out]
          n125 = Build Array(w362, w363, 0.0 ("element"), 0.0 ("element")) -> (w356:dbl[])
          n126 = Add(x=w356, y=w357) -> (x+y=w355:dbl[])
        }
      }
      event "Bless from OGP": Value Change {
        # "center of lower module"
        # "center of upper module"
        # "NL line with correct rotation"
        # "center of lower module"
        # "center of upper module"
        # "Default stave dimension\namong mounting holes"
        # "Measure 2 module positions on stave"
        n127 = event-data() -> ()  [unwired: 1 in, 6 out]
        n128 = Build Array(34.0 ("element"), 470.0 ("element"), 0.0 ("element"), 0.0 ("element")) -> ()  [unwired: 1 out]
        n129 = for {
          N: 1 -> [_]
          tunnel: w415 -> [_]
          shift-right: [w452] -> w414
          shift-left: w388 -> [w465]
          tunnel: w390 -> [_]
          tunnel: [w444] -> w393
          tunnel: [w447] -> w401
          tunnel: w389 -> [w454]
          tunnel: [w430] -> w374
          (unwired) FALSE ("Inital GO")
          (unwired) "ideal delta Y between \n2 fiducial marks"
          (unwired) "ideal delta X between 2 fiducial marks"
          # "after NL"
          # "after SL"
          # "NL line"
          # "rotation"
          n130 = call "Joystick and Camera SHIH VPC- external Connection.vi"("Motion in"=w465, "XYZTheta"=dbl[] [587.6501861346682, 659.8354057217969, 70.1155335060548, 0.010000094994154989] ("N chip"), "Measurement Point"="north chip", "Inital GO"=TRUE) -> ("Motion out"=w462:refnum<class "Motion.lvclass">, "Sum"=w442:dbl[])  [unwired: 3 in, 2 out]
          "N chip" <- w442
          n131 = call "Joystick and Camera SHIH VPC- external Connection.vi"("Motion in"=w462, "XYZTheta"=dbl[] [614.8404990206996, 1158.7590823829282, 70.34521582498871, 0.010000670236950445] ("S chip"), "Measurement Point"="south chip", "Inital GO"=TRUE) -> ("Motion out"=w461:refnum<class "Motion.lvclass">, "Sum"=w443:dbl[])  [unwired: 3 in, 2 out]
          "S chip" <- w443
          n132 = Subtract(x=w443, y=w442) -> (x-y=w441:dbl[])
          n133 = Index Array(array=w441, index #1=0 ("index"), index #2=1 ("index")) -> (element #1=w438:dbl, element #2=w437:dbl)
          n134 = Square(x=w438) -> (x^2=w435:dbl)
          n135 = Square(x=w437) -> (x^2=w436:dbl)
          n136 = Add(x=w435, y=w436) -> (x+y=w434:dbl)
          n137 = call "Joystick and Camera SHIH VPC- external Connection.vi"("Motion in"=w461, "Measurement Point"="height of stave", "Inital GO"=FALSE) -> ("Motion out"=w452:refnum<class "Motion.lvclass">, "Sum"=w453:dbl[])  [unwired: 4 in, 2 out]
          n138 = call "O to G peek.vi"("height"=w453, "south chip"=w443, "north chip"=w442, "Input file"=w454) -> ("OGP length"=→"chip distance by OGP":dbl, "output BR"=w456:dbl[], "output BL"=w455:dbl[], "output TL"=w449:dbl[])  [unwired: 4 in]
          "after NL" <- w449
          "after SR" <- w456
          "after SL" <- w455
          n139 = Square Root(x=w434) -> (sqrt(x)=→"chip distance by gantry":dbl)
          n140 = Subtract(x=w456, y=w449) -> (x-y=w467:dbl[])
          n141 = Build Array(24.3 ("y"), 231.4 ("y"), 0.0 ("element"), -0.05 ("element")) -> ()  [unwired: 1 out]
          n142 = Subtract(x=w455, y=w449) -> (x-y=w473:dbl[])
          n143 = call "XY_to_Rotation_RPHI.vi"("X-Y"=w473) -> ("r-phi"=w472:dbl[])
          n144 = Index Array(array=w472, index=1) -> (element=w469:dbl)
          n145 = Multiply(x=w469, y=-1.0) -> (x*y=w447:dbl)
          n146 = Replace Array Subset(array=w467, new element=w447, index=3) -> (→"bless from OGP !! measured stave size":dbl[])
          n147 = Replace Array Subset(array=w449, new element=w447, index=3) -> (w445:dbl[])
          n148 = Add(x=w456, y=w449) -> (x+y=w479:dbl[])
          n149 = Divide(x=w479, y=2.0) -> (x/y=w431:dbl[])
          n150 = Add(x=w445, y=dbl[] [0.0, 10.0, 0.0, 0.0]) -> (x+y=w444:dbl[])
          n151 = Replace Array Subset(array=w431, new element=w447, index=3) -> (w430:dbl[])
          "bless from OGP !!! Center of  stave" <- w430
        }
        n152 = Build Array(0.0 ("element"), 238.0 ("element"), 0.0 ("element"), 0.0 ("element")) -> (w394:dbl[])
        n153 = Add(x=w393, y=w394) -> (x+y=w392:dbl[])
        n154 = Build Array(w393, w392) -> (w391:dbl[][])
        n155 = Build Array(0.0 ("element"), 116.65 ("element"), 0.0 ("element"), 0.0 ("element")) -> (w375:dbl[])
        n156 = Build Array(0.0 ("element"), -116.65 ("element"), 0.0 ("element"), 0.0 ("element")) -> (w376:dbl[])
        n157 = Build Array(17.0 ("element"), 411.0 ("element"), 0.0 ("element"), 0.0 ("element")) -> (w402:dbl[])
        n158 = Build Array(17.0 ("element"), 60.9 ("element"), 0.0 ("element"), 0.0 ("element")) -> (w403:dbl[])
        n159 = case shown="True" w385 {
          tunnel: w376 -> [w426 w429]
          tunnel: w375 -> [w425 w428]
          tunnel: [w424 w427] -> w373
          frame False {
            n160 = Build Array(w425, w426) -> (w424:dbl[][])
          }
          frame True {
            n161 = Build Array(w429, w428) -> (w427:dbl[][])
          }
        }
        n162 = case shown="True" w385 {
          tunnel: w403 -> [w498 w501]
          tunnel: w402 -> [w497 w500]
          tunnel: [w496 w499] -> _
          frame False {
            n163 = Build Array(w497, w498) -> (w496:dbl[][])
          }
          frame True {
            n164 = Build Array(w501, w500) -> (w499:dbl[][])
          }
        }
        n165 = for {
          tunnel: w373 -> [w489] mode=indexing
          tunnel: w401 -> [w486]
          tunnel: [w488] -> w387 mode=indexing
          tunnel: w374 -> [w482]
          tunnel: [w481] -> w372 mode=indexing
          n166 = Multiply(x=w486, y=-1.0) -> (x*y=w485:dbl)
          n167 = Index Array(array=w489, index=0) -> (element=w492:dbl)
          n168 = Index Array(array=w489, index=1) -> (element=w491:dbl)
          n169 = call-poly <vilib>:"2D Cartesian Coordinate Rotation.vi"("theta"=w485, "y"=w491, "x"=w492) -> ("y out"=w494:dbl, "x out"=w493:dbl)  [unwired: 6 in, 1 out]
          n170 = Build Array(w493, w494, 0.0 ("element"), 0.0 ("element")) -> (w481:dbl[])
          n171 = Add(x=w481, y=w482) -> (x+y=w488:dbl[])
        }
        "HPoS_CT" <- w372
        n172 = Add(x=w387, y=w371) -> (x+y=w386:dbl[][])
      }
      event "Measure Pickup Tools": Value Change {
        (unwired) "Measuring Pickup Tools" ("String")
        n173 = event-data() -> ()  [unwired: 1 in, 6 out]
        n174 = for {
          N: w504 -> [_]
          tunnel: [w537] -> w512 mode=indexing
          tunnel: w513 -> [w541]
          tunnel: [w523] -> w511
          tunnel: w510 -> [w522] mode=indexing
          # "Default size and\norientation"
          n175 = call "Joystick and Camera SHIH VPC- external Connection.vi"("Motion in"=w541, "XYZTheta"=w522, "Measurement Point"="PickUp tool Top") -> ("Motion out"=w517:refnum<class "Motion.lvclass">, "Sum"=w540:dbl[])  [unwired: 4 in, 2 out]
          n176 = Build Array(0.0 ("element"), 29.94 ("element"), 0.0 ("element"), 0.0 ("element")) -> (w528:dbl[])
          n177 = Add(x=w540, y=w528) -> (x+y=w514:dbl[])
          n178 = Array Subset(array=w514, index=0, length=2) -> (w515:dbl[])
          n179 = call-dynamic "XY Go.vi"("Speed"=20.0, "XY"=w515, "Motion in"=w517) -> ("Motion out"=w516:refnum<class "Motion.lvclass">)  [unwired: 7 in, 1 out]
          n180 = call "Joystick and Camera SHIH VPC- external Connection.vi"("Motion in"=w516, "Measurement Point"="PickUp tool Bottom", "Inital GO"=FALSE) -> ("Motion out"=w523:refnum<class "Motion.lvclass">, "Sum"=w539:dbl[])  [unwired: 4 in, 2 out]
          n181 = Add(x=w540, y=w539) -> (x+y=w546:dbl[])
          n182 = Subtract(x=w539, y=w540) -> (x-y=w538:dbl[])
          n183 = Divide(x=w546, y=2.0) -> (x/y=w543:dbl[])
          n184 = call "XYtoRPHI.vi"("X-Y"=w538) -> ("r-phi"=w544:dbl[])
          n185 = Index Array(array=w544, index=1) -> (element=w532:dbl)
          n186 = Absolute Value(x=w532) -> (abs(x)=w535:dbl)
          n187 = Sign(1:w532) -> (0:w533:dbl)
          n188 = Subtract(x=w535, y=1.5707963267948966) -> (x-y=w534:dbl)
          n189 = Multiply(x=w533, y=w534) -> (x*y=w531:dbl)
          n190 = Replace Array Subset(array=w543, new element=w531, index=3) -> (w537:dbl[])
          "PickupTool \nCenterPosition" <- w537
        }
      }
      event "Deposit Glue": Value Change {
        # "CF height"
        # "surface z offset"
        # "two sensor, Sensor B then A"
        # "Unmount syringe"
        # "first needle park position\nneedle gap on Z value : 0.5 mm"
        # "Syringe-camera offset"
        n191 = event-data() -> ()  [unwired: 1 in, 6 out]
        n192 = call-poly <vilib>:"Read Delimited Spreadsheet.vi"("file path (dialog if empty)"=path "D:/INTT/V1/Assembly Data/Tool Offsets/Dispense Tip Offset.txt", "number of rows (all:-1)"=-1) -> ("first row"=w602:dbl[])  [unwired: 8 in, 5 out]
        n193 = Add(x=14.2 ("element"), y=w558) -> (x+y=w552:dbl)
        n194 = Index Array(array=w602, index #1=0 ("index"), index #2=1 ("index")) -> (element #1=w597:dbl, element #2=w595:dbl)
        n195 = Build Array(w597, w595, 0.0 ("element"), 0.0 ("element")) -> (w581:dbl[])
        n196 = Array Subset(array=w548, index (row)=0, length (row)=1 ("length")) -> (w561:dbl[][])  [unwired: 2 in]
        n197 = Reshape Array(w561, 4 ("dimension size")) -> (w554:dbl[])
        n198 = Index Array(array=w554, index=2) -> (element=w549:dbl)
        n199 = Add(x=w549, y=w552) -> (x+y=w551:dbl)
        n200 = Build Array(436.638, 1040.76, w551, 0.0 ("element")) -> (w550:dbl[])
        "Needle parking position" <- w550
        n201 = call "XYZTheta Go.vi"("XYZTheta In"=w550, "Motion in"=w586) -> ("error out"=w594:errorcluster, "Motion out"=w585:refnum<class "Motion.lvclass">)  [unwired: 7 in, 1 out]
        n202 = call "Display Message to User"("error in (no error)"=w594) -> ("error out"=w587:errorcluster)  [unwired: 9 in, 1 out]
        n203 = case shown="False" w556 {
          tunnel: w548 -> [w610 w619]
          tunnel: [w607 w619] -> w555
          frame False {
            n204 = Array Subset(array=w610, index (row)=1 ("index"), length (row)=1 ("length")) -> (w611:dbl[][])  [unwired: 2 in]
            n205 = Array Subset(array=w610, index (row)=0 ("index"), length (row)=1 ("length")) -> (w614:dbl[][])  [unwired: 2 in]
            n206 = Reshape Array(w614, 4 ("dimension size")) -> (w609:dbl[])
            n207 = Reshape Array(w611, 4 ("dimension size")) -> (w608:dbl[])
            n208 = Build Array(w608, w609) -> (w607:dbl[][])
          }
          frame True {
          }
        }
        n209 = call-dynamic "Z Go.vi"("error in (no error)"=w587, "Speed"=20.0, "Position"=0.0, "Motion in"=w585) -> ("error out"=w584:errorcluster, "Motion out"=w590:refnum<class "Motion.lvclass">)  [unwired: 6 in]
        n210 = call "Display Message to User2"("error in (no error)"=w584) -> ("error out"=w583:errorcluster)  [unwired: 9 in, 1 out]
        n211 = Add(x=w549, y=-2.5) -> (x+y=w591:dbl)
        n212 = call-dynamic "Z Go.vi"("error in (no error)"=w583, "Speed"=20.0, "Position"=w591, "Motion in"=w590) -> ("error out"=w560:errorcluster, "Motion out"=w582:refnum<class "Motion.lvclass">)  [unwired: 6 in]
        n213 = call-dynamic "Connect.vi"("Ultimus V in"=refnum<class "Ultimus V2.lvclass"> refnum ("Ultimus V2.lvclass")) -> ("Ultimus V out"=w580:refnum<class "Ultimus V2.lvclass">)  [unwired: 9 in, 1 out]
        n214 = for {
          N: w575 -> [_]
          tunnel: w582 -> [w634]
          tunnel: w580 -> [w633]
          tunnel: w581 -> [w635]
          tunnel: w570 -> [_] mode=indexing
          tunnel: w555 -> [w636] mode=indexing
          tunnel: [w632] -> w568
          tunnel: [w631] -> w567
          tunnel: w560 -> [w627]
          tunnel: [w628] -> w559
          tunnel: w557 -> [w626]
          (unwired) 100.0 ("Speed")
          n215 = Add(x=w636, y=w635) -> (x+y=w666:dbl[])
          n216 = Add(x=w666, y=dbl[] [3.3, 5.0, 0.0, 0.0]) -> (x+y=w667:dbl[])
          n217 = Index Array(array=w667, index=2) -> (element=w624:dbl)
          n218 = Array Subset(array=w667, index=0, length=2) -> (w642:dbl[])
          n219 = call-dynamic "XY Go.vi"("error in (no error)"=w627, "Speed"=100.0, "XY"=w642, "Motion in"=w634) -> ("error out"=w622:errorcluster, "Motion out"=w623:refnum<class "Motion.lvclass">)  [unwired: 6 in]
          n220 = case shown="True" "check height?" {
            tunnel: w624 -> [_ w683]
            tunnel: w623 -> [w676 w682]
            tunnel: w622 -> [w677 w681]
            tunnel: [w677 w679] -> w621
            tunnel: [w676 w678] -> w620
            frame False {
            }
            frame True {
              n221 = call-dynamic "Z Go.vi"("error in (no error)"=w681, "Speed"=5.0, "Position"=w683, "Motion in"=w682) -> ("error out"=w680:errorcluster, "Motion out"=w678:refnum<class "Motion.lvclass">)  [unwired: 6 in]
              n222 = call "Display Message to User4"("error in (no error)"=w680) -> ("error out"=w679:errorcluster)  [unwired: 9 in, 1 out]
            }
          }
          n223 = Add(x=w624, y=-2.0) -> (x+y=w641:dbl)
          n224 = call-dynamic "Z Go.vi"("error in (no error)"=w621, "Speed"=5.0, "Position"=w641, "Motion in"=w620) -> ("error out"=w639:errorcluster, "Motion out"=w640:refnum<class "Motion.lvclass">)  [unwired: 6 in]
          n225 = call "Muliti_XY_dispense.vi"("Pressure"=w626, "Path count"=4, "distances"=dbl[][] [[0.0, 224.0], [27.4, 0.0], [0.0, -224.0], [-27.4, 0.0]], "Ultimus V in"=w633, "Motion in"=w640) -> ("Ultimus V out"=w660:refnum<class "Ultimus V2.lvclass">, "Motion out"=w665:refnum<class "Motion.lvclass">)  [unwired: 5 in]
          n226 = call-dynamic "wrtCurrent Go.vi"("axis names"=string[] ["X", "Y"], "error in (no error)"=w639, "Speed"=5.0, "distances"=dbl[] [4.6, 5.0], "Motion in"=w665) -> ("error out"=w630:errorcluster, "Motion out"=w659:refnum<class "Motion.lvclass">)  [unwired: 5 in]
          n227 = call "Muliti_XY_dispense.vi"("Pressure"=w626, "Path count"=4, "distances"=dbl[][] [[0.0, 214.0], [18.2, 0.0], [0.0, -214.0], [-18.2, 0.0]], "Ultimus V in"=w660, "Motion in"=w659) -> ("Ultimus V out"=w652:refnum<class "Ultimus V2.lvclass">, "Motion out"=w651:refnum<class "Motion.lvclass">)  [unwired: 5 in]
          n228 = call-dynamic "wrtCurrent Go.vi"("axis names"=string[] ["X", "Y"], "error in (no error)"=w630, "Speed"=5.0, "distances"=dbl[] [4.6, 5.0], "Motion in"=w651) -> ("error out"=w629:errorcluster, "Motion out"=w650:refnum<class "Motion.lvclass">)  [unwired: 5 in]
          n229 = call "Muliti_XY_dispense.vi"("Pressure"=w626, "Path count"=4, "distances"=dbl[][] [[0.0, 204.0], [9.0, 0.0], [0.0, -204.0], [-9.0, 0.0]], "Ultimus V in"=w652, "Motion in"=w650) -> ("Ultimus V out"=w637:refnum<class "Ultimus V2.lvclass">, "Motion out"=w638:refnum<class "Motion.lvclass">)  [unwired: 5 in]
          n230 = call-dynamic "wrtCurrent Go.vi"("axis names"=string[] ["X", "Y"], "error in (no error)"=w629, "Speed"=5.0, "distances"=dbl[] [4.5, 5.0], "Motion in"=w638) -> ("error out"=w628:errorcluster, "Motion out"=w644:refnum<class "Motion.lvclass">)  [unwired: 5 in]
          n231 = call "Muliti_XY_dispense.vi"("Pressure"=w626, "Path count"=1, "distances"=dbl[][] [[0.0, 194.0], [7.0, 0.0], [0.0, -206.0], [-7.0, 0.0]], "Ultimus V in"=w637, "Motion in"=w644) -> ("Ultimus V out"=w631:refnum<class "Ultimus V2.lvclass">, "Motion out"=w632:refnum<class "Motion.lvclass">)  [unwired: 5 in]
        }
        n232 = call "XYZTheta Go.vi"("error in (no error)"=w559, "XYZTheta In"=dbl[] [500.0, 1000.0, 0.0, 0.1], "Motion in"=w568) -> ("error out"=w578:errorcluster, "Motion out"=w576:refnum<class "Motion.lvclass">)  [unwired: 6 in, 1 out]
        n233 = call "Display Message to User3"("error in (no error)"=w578) -> ()  [unwired: 9 in, 2 out]
        n234 = call-dynamic "Disconnect.vi"("Ultimus V in"=w567) -> ()  [unwired: 9 in, 1 out]
      }
      event "Needle Alignment": Value Change {
        (unwired) "Needle Alignment in progress ...." ("String")
        # "CF height"
        # "surface z offset"
        # "first needle park position\nneedle gap on Z value : 0.5 mm"
        # "Syringe-camera offset"
        n235 = event-data() -> ()  [unwired: 1 in, 6 out]
        n236 = Array Subset(array=w686, index (row)=0, length (row)=1 ("length")) -> (w689:dbl[][])  [unwired: 2 in]
        n237 = Reshape Array(w689, 4 ("dimension size")) -> (w688:dbl[])
        n238 = Index Array(array=w688, index=2) -> (element=w685:dbl)
        n239 = call-poly <vilib>:"Read Delimited Spreadsheet.vi"("file path (dialog if empty)"=path "D:/INTT/V1/Assembly Data/Tool Offsets/Dispense Tip Offset.txt", "number of rows (all:-1)"=-1) -> ("first row"=w736:dbl[])  [unwired: 8 in, 5 out]
        n240 = Index Array(array=w736, index #1=0 ("index"), index #2=1 ("index")) -> (element #1=w731:dbl, element #2=w730:dbl)
        n241 = Add(x=14.2 ("element"), y=w694) -> (x+y=w696:dbl)
        n242 = Add(x=w685, y=w696) -> (x+y=w695:dbl)
        n243 = Build Array(436.638, 1040.76, w695, 0.0 ("element")) -> (w693:dbl[])
        n244 = Build Array(w731, w730, 0.0 ("element"), 0.0 ("element")) -> (w705:dbl[])
        n245 = call "XYZTheta Go.vi"("XYZTheta In"=w693, "Motion in"=w720) -> ("error out"=w729:errorcluster, "XYZTheta Out"=w710:dbl[], "Motion out"=w719:refnum<class "Motion.lvclass">)  [unwired: 7 in]
        n246 = call "Display Message to User10"("error in (no error)"=w729) -> ("error out"=w726:errorcluster)  [unwired: 9 in, 1 out]
        n247 = call-dynamic "Z Go.vi"("error in (no error)"=w726, "Speed"=20.0, "Position"=0.0, "Motion in"=w719) -> ("Motion out"=w718:refnum<class "Motion.lvclass">)  [unwired: 6 in, 1 out]
        n248 = Replace Array Subset(array=w710, new element=0.0 ("new element/subarray"), index=2) -> (w707:dbl[])
        n249 = call "Joystick and Camera - external Connection.vi"("Motion in"=w718, "XYZTheta"=w707, "Measurement Point"="Touch Needle on a surface") -> ("Motion out"=w716:refnum<class "Motion.lvclass">, "Gantry"=w706:dbl[])  [unwired: 4 in, 2 out]
        n250 = Subtract(x=w706, y=w705) -> (x-y=w704:dbl[])
        n251 = call "Joystick and Camera - external Connection.vi"("Motion in"=w716, "XYZTheta"=w704, "Measurement Point"="Measure the touch spot with camera") -> ("Motion out"=w712:refnum<class "Motion.lvclass">, "Gantry"=w715:dbl[])  [unwired: 4 in, 2 out]
        n252 = Subtract(x=w706, y=w715) -> (x-y=w714:dbl[])
        n253 = call-poly <vilib>:"Write Delimited Spreadsheet.vi"("file path (dialog if empty)"=path "D:/INTT/V1/Assembly Data/Tool Offsets/Dispense Tip Offset.txt", "1D data"=w714, "append to file? (new file:F)"=FALSE) -> ()  [unwired: 11 in, 2 out]
      }
      event "Pick and place": Value Change {
        (unwired) "PICK and PLACE samples ..." ("String")
        n254 = event-data() -> ()  [unwired: 1 in, 6 out]
        n255 = case shown="True" w742 {
          tunnel: w745 -> [w869 w891]
          tunnel: [w868 w890] -> w744
          frame False {
            n256 = Array Subset(array=w869, index (row)=0 ("index"), length (row)=1 ("length")) -> (w871:dbl[][])  [unwired: 2 in]
            n257 = Build Array(11.75 ("element"), 173.55 ("element"), 0.0 ("element"), 0.0 ("element")) -> (w875:dbl[])
            n258 = Reshape Array(w871, 4 ("dimension size")) -> (w870:dbl[])
            n259 = Add(x=w875, y=w870) -> (x+y=w868:dbl[])
          }
          frame True {
            n260 = Array Subset(array=w891, index (row)=0 ("index"), length (row)=1 ("length")) -> (w881:dbl[][])  [unwired: 2 in]
            n261 = Build Array(11.75 ("element"), 56.85 ("element"), 0.0 ("element"), 0.0 ("element")) -> (w885:dbl[])
            n262 = Reshape Array(w881, 4 ("dimension size")) -> (w880:dbl[])
            n263 = Add(x=w885, y=w880) -> (x+y=w890:dbl[])
          }
        }
        n264 = call-poly <vilib>:"Read Delimited Spreadsheet.vi"("file path (dialog if empty)"=path "D:/INTT/V1/Assembly Data/Tool Offsets/Bellows Tool Offset.txt", "number of rows (all:-1)"=-1) -> ("first row"=w761:dbl[])  [unwired: 8 in, 5 out]
        n265 = Index Array(array=w761, index #1=0 ("index"), index #2=1 ("index"), index #3=2 ("index")) -> (element #1=w757:dbl, element #2=w756:dbl, element #3=w755:dbl)
        n266 = for {
          N: 1 -> [_]
          tunnel: w764 -> [w773]
          tunnel: [w794] -> w754
          tunnel: w753 -> [w766] mode=indexing
          tunnel: [w782] -> w748
          tunnel: w749 -> [w772]
          tunnel: w757 -> [w796]
          tunnel: w756 -> [w795]
          tunnel: w755 -> [w793]
          tunnel: w750 -> [w788]
          tunnel: w747 -> [w775]
          tunnel: w744 -> [w774]
          tunnel: w740 -> [w770]
          tunnel: w741 -> [w765]
          w784 = 0 ("Write")
          w787 = TRUE ("Write Value")
          # "putback pickup tool"
          # "pickup tool"
          # "pickup tool height offset"
          # "Pick up PICKUP TOOL"
          # "Pick up CHIPs/Sensor and place on HDI"
          n267 = Build Array(w796, w795, w793, 0.0 ("element")) -> (w767:dbl[])
          n268 = Add(x=w766, y=w767) -> (x+y=w768:dbl[])
          n269 = call "XYZTheta-2Zspeed Go.vi"("XYZTheta In"=w768, "Motion in"=w773) -> ("error out"=w771:errorcluster, "Motion out"=w769:refnum<class "Motion.lvclass">)  [unwired: 7 in, 1 out]
          n270 = call "WriteReadWait.vi"("Read Value"=w787, "Write Value"=w787, "error in (no error)"=w771, "Read"=w784, "Write"=w784, "I-O in"=w772) -> ("error out"=w786:errorcluster, "I-O out"=w785:refnum<class "NI-DAQ.lvclass">)  [unwired: 4 in]
          n271 = Replace Array Subset(array=w767, new element=-16.0 ("t"), index=2) -> (w791:dbl[])
          n272 = for {
            N: w788 -> [_]
            tunnel: w769 -> [w815]
            tunnel: w791 -> [w814]
            tunnel: w786 -> [w813]
            tunnel: [w812] -> w797
            tunnel: w785 -> [w811]
            tunnel: [w810] -> w783
            tunnel: [w809] -> w790
            tunnel: w775 -> [w806]
            tunnel: w774 -> [w805]
            tunnel: w770 -> [w804] mode=indexing
            tunnel: w765 -> [w803] mode=indexing
            n273 = flat-sequence {
              tunnel: [w835] -> w816
              tunnel: w815 -> [w834]
              tunnel: w814 -> [w833]
              tunnel: w813 -> [w831]
              tunnel: w811 -> [w823]
              tunnel: [w830] -> w808
              tunnel: [w827] -> w807
              tunnel: w806 -> [w820]
              tunnel: w805 -> [w826]
              tunnel: w816 -> [w855]
              tunnel: [w867] -> w812
              tunnel: [w866] -> _
              tunnel: w814 -> [_]
              tunnel: [w862] -> w810
              tunnel: [w859] -> w809
              tunnel: w808 -> [w864]
              tunnel: w807 -> [w860]
              tunnel: w804 -> [w861]
              tunnel: w803 -> [w839]
              frame #0 {
                w821 = FALSE ("Write Value")
                w828 = TRUE ("Write Value")
                w829 = 1 ("Write")
                # "pickup module"
                # "release module"
                # "pickup sample from tray"
                n274 = Add(x=w826, y=w833) -> (x+y=w832:dbl[])
                n275 = call "XYZTheta-2Zspeed Go.vi"("error in (no error)"=w831, "XYZTheta In"=w832, "Motion in"=w834) -> ("error out"=w824:errorcluster, "Motion out"=w835:refnum<class "Motion.lvclass">)  [unwired: 6 in, 1 out]
                n276 = call "Time Delay"("error in (no error)"=w824) -> ("error out"=w817:errorcluster)  [unwired: 10 in]
                n277 = call "0"("error in (no error)"=w817) -> ("error out"=w818:errorcluster)  [unwired: 9 in, 1 out]
                n278 = call "WriteReadWait.vi"("Read Value"=w821, "Write Value"=w821, "error in (no error)"=w818, "Read"=w820, "Write"=w820, "I-O in"=w823) -> ("error out"=w819:errorcluster, "I-O out"=w822:refnum<class "NI-DAQ.lvclass">)  [unwired: 4 in]
                n279 = call "Time Delay3"("error in (no error)"=w819) -> ("error out"=w825:errorcluster)  [unwired: 10 in]
                n280 = call "WriteReadWait.vi"("Read Value"=w828, "Write Value"=w828, "error in (no error)"=w825, "Read"=w829, "Write"=w829, "I-O in"=w822) -> ("error out"=w827:errorcluster, "I-O out"=w830:refnum<class "NI-DAQ.lvclass">)  [unwired: 4 in]
              }
              frame #1 {
                w863 = 1 ("Write")
                w865 = FALSE ("Write Value")
                # "lift for chip/sensor thickness"
                # "place sample on HDI"
                n281 = Add(x=w861, y=dbl[] [0.0, 0.0, -16.0, 0.0]) -> (x+y=w853:dbl[])
                n282 = call-dynamic "Get Current Position.vi"("Motion in"=w855) -> ("XYZTheta Out"=w851:dbl[], "Motion out"=w854:refnum<class "Motion.lvclass">)  [unwired: 8 in, 1 out]
                "gantry position test" <- w851
                n283 = Array Subset(array=w839, index=0, length=2) -> (w840:dbl[])
                n284 = Build Array (concatenate)(w840, 0.0 ("element"), 0.0 ("element")) -> (w838:dbl[])
                n285 = Subtract(x=w853, y=w838) -> (x-y=w852:dbl[])
                "displacement" <- w852
                n286 = Array Subset(array=w851, index=0, length=2) -> (w846:dbl[])
                n287 = Build Array (concatenate)(w846, 0.0 ("element"), 0.0 ("element")) -> (w845:dbl[])
                n288 = Add(x=w845, y=w852) -> (x+y=w837:dbl[])
                "stave target position" <- w837
                n289 = call "XYZTheta-2Zspeed Go.vi"("error in (no error)"=w860, "XYZTheta In"=w837, "Motion in"=w854) -> ("error out"=w858:errorcluster, "XYZTheta Out"=w866:dbl[], "Motion out"=w867:refnum<class "Motion.lvclass">)  [unwired: 6 in]
                n290 = call "1"("error in (no error)"=w858) -> ("error out"=w857:errorcluster)  [unwired: 9 in, 1 out]
                n291 = call "Time Delay6"("error in (no error)"=w857) -> ("error out"=w856:errorcluster)  [unwired: 10 in]
                n292 = call "WriteReadWait.vi"("Read Value"=w865, "Write Value"=w865, "error in (no error)"=w856, "Read"=w863, "Write"=w863, "I-O in"=w864) -> ("error out"=w859:errorcluster, "I-O out"=w862:refnum<class "NI-DAQ.lvclass">)  [unwired: 4 in]
              }
            }
          }
          n293 = call "XYZTheta-2Zspeed Go.vi"("error in (no error)"=w790, "XYZTheta In"=w768, "Motion in"=w797) -> ("error out"=w778:errorcluster, "Motion out"=w801:refnum<class "Motion.lvclass">)  [unwired: 6 in, 1 out]
          n294 = call "Time Delay9"("error in (no error)"=w778) -> ("error out"=w780:errorcluster)  [unwired: 10 in]
          n295 = call-dynamic "Digital Write 1 Channel.vi"("DAQ Module"=0, "error constant"=w780, "Value"=FALSE, "Channel"=0, "NI-DAQ.lvclass"=w783) -> ("error IO"=w779:errorcluster, "NI-DAQ.lvclass 2"=w782:refnum<class "NI-DAQ.lvclass">)  [unwired: 5 in]
          n296 = call "Time Delay10"("error in (no error)"=w779) -> ("error out"=w798:errorcluster)  [unwired: 10 in]
          n297 = call-dynamic "Z Go.vi"("error in (no error)"=w798, "Speed"=10.0, "Position"=0.0 ("new element/subarray"), "Motion in"=w801) -> ("Motion out"=w794:refnum<class "Motion.lvclass">)  [unwired: 6 in, 1 out]
        }
      }
      event "GOTO": Value Change {
        (unwired) "GOING to a position" ("String")
        n298 = event-data() -> ()  [unwired: 1 in, 6 out]
        n299 = call "XYZTheta Go.vi"("XYZTheta In"="Parking position", "Motion in"=w897) -> ("Motion out"=w895:refnum<class "Motion.lvclass">)  [unwired: 7 in, 2 out]
      }
      event "READ Position": Value Change {
        n300 = event-data() -> ()  [unwired: 1 in, 6 out]
        n301 = call-dynamic "Get Current Position.vi"("Motion in"=w915) -> ("XYZTheta Out"=→"Gantry current position":dbl[], "Motion out"=w914:refnum<class "Motion.lvclass">)  [unwired: 8 in, 1 out]
      }
      event "HDI vacuum": Value Change {
        n302 = event-data() -> ()  [unwired: 1 in, 6 out]
        n303 = call "WriteReadWait.vi"("Read Value"="vacuum", "Write Value"="vacuum", "Read"=w926, "Write"=w926, "I-O in"=w929) -> ("error out"=w927:errorcluster, "I-O out"=w916:refnum<class "NI-DAQ.lvclass">)  [unwired: 5 in]
        n304 = call "Time Delay2"("error in (no error)"=w927) -> ()  [unwired: 10 in, 1 out]
      }
      event Timeout {
        n305 = event-data() -> ()  [unwired: 1 in, 3 out]
        n306 = call-dynamic "Digital Read 1 Channel.vi"("Read"=w940, "NI-DAQ in"=w941) -> ("Value"=→"Status":bool, "NI-DAQ out"=w939:refnum<class "NI-DAQ.lvclass">)  [unwired: 7 in, 1 out]
      }
    }
    "Measured HDI size" <- w19
    "module positions on stave" <- w20
    "Stave mark" <- w18
    "measured HDI top-left position" <- w15
    n307 = feedback-in #1(w19) -> ()
    n308 = feedback-in #2(w18) -> ()
    n309 = feedback-in #3(w15) -> ()
    n310 = feedback-in #4(w31) -> ()
    n311 = feedback-in #5(w28) -> ()
    n312 = feedback-in #6(w36) -> ()
    n313 = feedback-in #7(w20) -> ()
    n314 = feedback-in #8(w37) -> ()
    "# of tasks excuted" <- w33
  }
  n315 = call-dynamic "Disconnect.vi"("Controller in"=w4) -> ()  [unwired: 9 in, 1 out]
  n316 = call-dynamic "Disconnect.vi"("I-O in"=w1) -> ()  [unwired: 9 in, 1 out]
